vi "Process_LogEngine.vi"(8 "error in (no error)":errorcluster, 9 "start process sync notifier":refnum<notifier>, 11 "LogEngine":refnum<class "LogEngine.lvclass">) -> (0 "error out":errorcluster)   [LabVIEW 2022 SP3, in "LogEngine.lvclass"]
doc: "Developed by Kevin Thompson\nkevin@thompsonengineering.net\n\nCopyright 2018-2020\nThompson Engineering, LLC"
uses:
  LogEngine.lvclass
  LogEngine.lvclass/LogEngine.ctl
  Support/DataQueues/DataQueues.lvclass
  Support/DataQueues/DataTypes/Analog DataSet MultiRow & ChanNames--cluster.ctl
  Support/DataQueues/DataTypes/Analog DataSet MultiRow & ChanNames--QRef.ctl
  Data Types/DAQ Q & TaskName--cluster.ctl
  Support/DataQueues/DataTypes/DataQ SelectType--enum.ctl
  Data Types/TD Logger State--enum.ctl
  Data Types/AsyncCmd_LogEngine--enum.ctl
  Data Types/TD Logger State Data--cluster.ctl
  Ichor_Common/Lib/ErrorHandler/ErrorHandler.lvclass
  <vilib>/TELLC/SMQ/Add States to Queue using MultiLine String with vData.vi
  DAQ/DAQ.lvclass
  Sequencer/Sequencer.lvclass
  Data Types/TD LogEngine LocalSMData--cluster.ctl
  DataTypes/SessionSettings--cluster.ctl
  Data Types/LogHeaderData--cluster.ctl
  Application/Application.lvclass
  Sequencer/DataTypes/LoadSeqStatus--enum.ctl
  DAQ/DataTypes/AsyncMsg_DAQ--enum.ctl
  DAQ/DataTypes/TD AI InstSettings--cluster.ctl
  Data Types/TD LogEngine Settings--cluster.ctl
  Sequencer/DataTypes/LoadSeqStatus EvData--cluster.ctl
panel:
  in  "localData":cluster{"Msg":string, "vData":variant}
  in  "Stop Process":bool
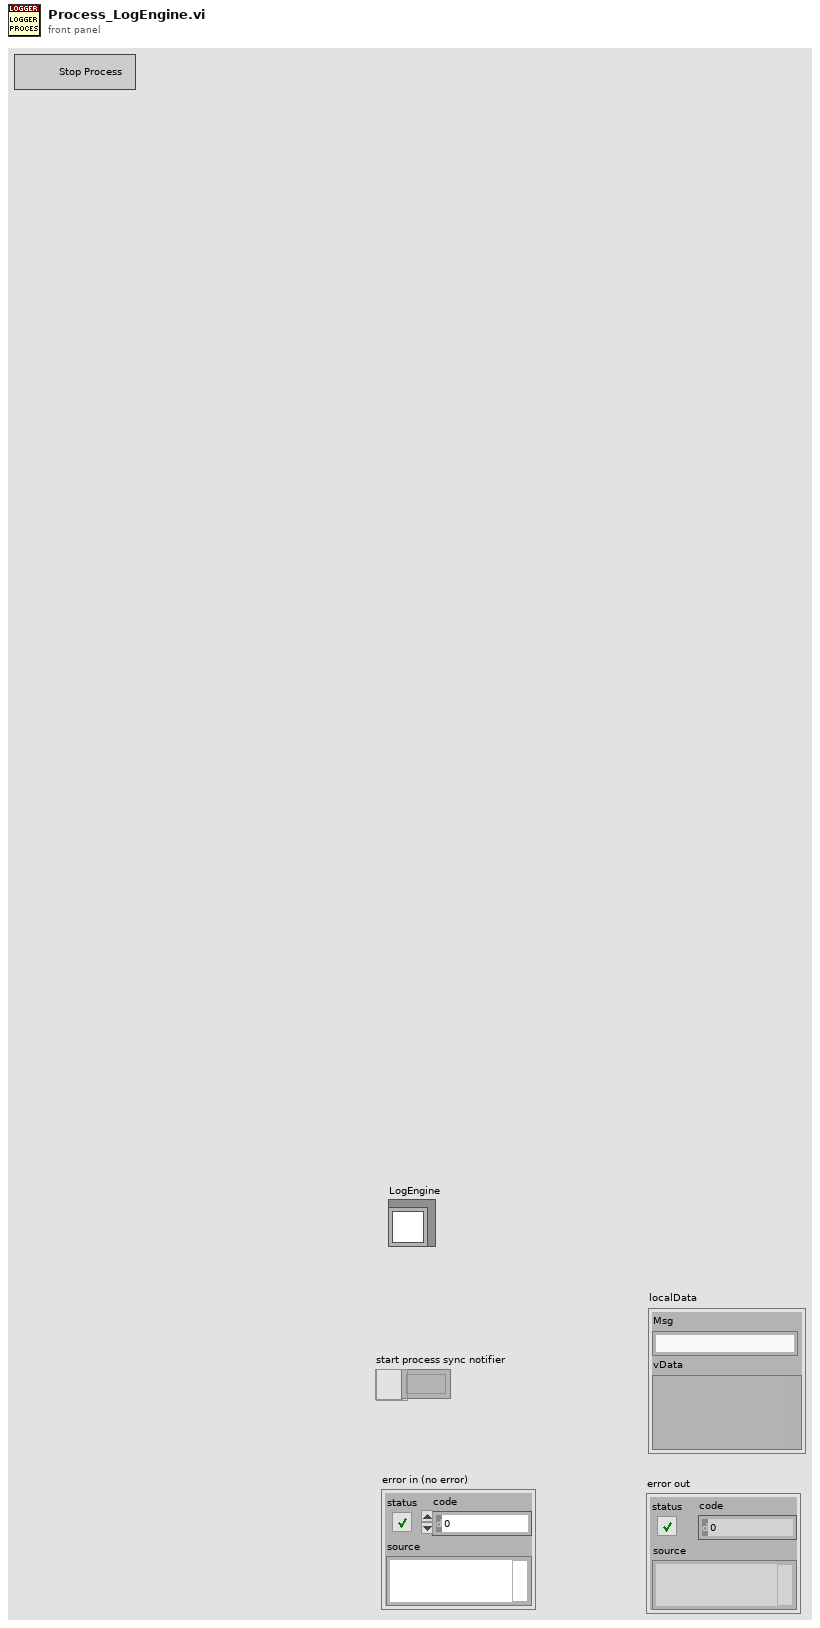
[diagram p1: front panel]
types:
  T1 = typedef "LogEngine.lvclass/TD LogEngine LocalSMData--cluster.ctl" = cluster{"Logging":bool, "tdms fileref":refnum<k34>, "Sequence File Path":string, "DAQ RawData Q []":T2[], "SMQ":refnum<queue>, "Core":cluster{"Current VI Ref":refnum<vi>, "process sync notifier":refnum<notifier>}, "quitting":bool, "Self Reference":refnum<class "LogEngine.lvclass">, "DAQ":refnum<class "DAQ.lvclass">, "TDMS file pathname":path, "Sequencer":refnum<class "Sequencer.lvclass">, "LogHeaderData":T4, "Application":refnum<class "Application.lvclass">, "dt(s)":dbl, "LogFile pathname":path, "LogEngine Settings":T6, "LogFile folder":path, "TDMS folder":path, "Logger State Data":T7, "TDMSLogging":bool, "HeaderStr Created?":bool, "TDMS SMQ":refnum<queue>, "StatusStr Ref":refnum<vi>, "Sampling dt(s)":dbl}
  T2 = typedef "LogEngine.lvclass/DAQ Q & TaskName--cluster.ctl" = cluster{"TaskName":string, "DAQ RawData Q":T3}
  T3 = typedef "DataQueues.lvclass/Analog DataSet MultiRow & ChanNames--QRef.ctl" = refnum<queue>
  T4 = typedef "LogEngine.lvclass/LogHeaderData--cluster.ctl" = cluster{"SessionSettings":T5, "SequenceFile":string, "Curr_WeldCount":i32, "AI TaskName":string, "SamplingRate":dbl, "SamplesPerAcq":i32}
  T5 = typedef "SessionSettings--cluster.ctl" = cluster{"Job_ID":string, "Operator_ID":string, "Station_ID":string, "Job_Description":string}
  T6 = typedef "LogEngine.lvclass/TD LogEngine Settings--cluster.ctl" = cluster{"placeholder":string, "LogWriteIntv (ms)":u32, "LogFile folder name":string, "TDMS folder name":string}
  T7 = typedef "LogEngine.lvclass/TD Logger State Data--cluster.ctl" = cluster{"Logger State":T8, "TDMS Logging State":T8, "LogFile path":path, "TDMS File path":path, "vData":variant}
  T8 = typedef "LogEngine.lvclass/TD Logger State--enum.ctl" = enum16{"Unknown", "Logging", "NotLogging", "Error"}
  T9 = typedef "DataQueues.lvclass/DataQ SelectType--enum.ctl" = enum16{"MainProcess", "LogEngine", "LocalDAQThread"}
  T10 = typedef "TD Pathnames--cluster.ctl" = cluster{"RunTimeSys?":bool, "AppFolder":path, "ExecutablePath":path, "ConfigFolder":path, "DataLogFolder":path, "SystemLogFolder":path, "SeqFolder":path, "MainStartupPathname":path, "MainUIPathname":path, "SystemEventsFile":path, "SeqEventsFile":path, "Config SettingsFile":path, "DAQ IOConfigFile":path, "SystemSimulation":bool}
  T11 = typedef "Sequencer.lvclass/LoadSeqStatus EvData--cluster.ctl" = cluster{"Time Stamp":timestamp, "OLD Status":T12, "NEW Status":T12}
  T12 = typedef "Sequencer.lvclass/LoadSeqStatus--enum.ctl" = enum16{"Unknown", "InProgress", "Loaded", "Failed"}
  T13 = typedef "DAQ.lvclass/AsyncMsg_DAQ--enum.ctl" = enum16{"DAQ.SendAI_InstSettings"}
  T14 = typedef "LogEngine.lvclass/AsyncCmd_LogEngine--enum.ctl" = enum16{"LE.CreateLogFile", "LE.EnableLogging", "LE.OpenTDMS", "LE.CloseTDMS", "LE.StartTDMSLogging", "LE.StopTDMSLogging", "LE.AppendStrToLog", "LE.ClearLogFilePathname"}
  T15 = typedef "Application.lvclass/AsynMsg_Application--enum.ctl" = enum16{"Application.AppClassReference", "Application.RefreshSettings", "Application.SendSessionSettings"}
  T16 = typedef "LogEngine.lvclass/TD Obj Data_LogEngine.ctl" = cluster{"LogEngine Settings":T6, "Logger State Data":T7, "tdms fileref":refnum<k34>, "LogHeaderData":T4, "LogHeaderString":string}
  T17 = typedef "Sequencer.lvclass/AsynMsg_Sequencer--enum.ctl" = enum16{"Sequencer.LoadSeqStatusChg", "Sequencer.SeqExecStatusChg", "Sequencer.SeqStepChg"}
  T18 = typedef "DAQ.lvclass/TD AI InstSettings--cluster.ctl" = cluster{"DaqRate":dbl, "NumSamples":i32}
  T19 = cluster{"AI InstSettings":T18, "AI TaskName":string}
  T20 = cluster{"dup Directory Path":path, "dup Directory Path":path}
  T21 = typedef "DAQ.lvclass/TD AI Instrument Settings--cluster.ctl" = cluster{"Disable":bool, "AI TaskName":string, "AI InstSettings":T18, "SimAI Ranges":T22}
  T22 = typedef "DAQ.lvclass/TD SimAI Ranges--cluster.ctl" = cluster{"lo":dbl, "hi":dbl}
  T23 = typedef "LogEngine.lvclass/TD LogEngine PublicEvents--cluster.ctl" = cluster{"stop process":refnum<user-event>, "LogEngine.AsyncCmd Event":refnum<user-event>, "LogEngine.AsyncMsg Event":refnum<user-event>, "Logger StateChanged Event":refnum<user-event>}
  T24 = typedef "Application.lvclass/Public Events--cluster.ctl" = cluster{"Application.AsyncCmd Event":refnum<user-event>, "Application.AsyncMsg Event":refnum<user-event>, "stop process":refnum<user-event>, "Application.ControlStateChg Event":refnum<user-event>, "Application.RadialGraph Event":refnum<user-event>}
  T25 = typedef "Sequencer.lvclass/Public Events--cluster.ctl" = cluster{"Sequencer.AsyncCmd Event":refnum<user-event>, "Sequencer.AsyncMsg Event":refnum<user-event>, "stop process":refnum<user-event>}
  T26 = typedef "DAQ.lvclass/TD PublicEvents--cluster.ctl" = cluster{"DaqOutputCmd Ev":refnum<user-event>, "stop process":refnum<user-event>, "DAQ.AsyncCmd Event":refnum<user-event>, "DAQStateChanged Event":refnum<user-event>, "DAQ.AsyncMsg Event":refnum<user-event>}
  T27 = cluster{bool, "Logger State Data":T7, "LogFile pathname":path}
  T28 = enum16{"open", "open or create", "create or replace", "create", "open (read-only)"}
  T29 = cluster{bool, "Logger State Data":T7, "TDMS file pathname":path}
  T30 = cluster{string, cluster{bool, "Logger State Data":T7, "TDMS file pathname":path}}
  T31 = cluster{string, cluster{bool, "Logger State Data":T7, path}}
  T32 = cluster{"Actuator ID":string[], "Cap":dbl[], "DF":dbl[], "Parameter":string[], "Parameter label":string, "Notes":string}
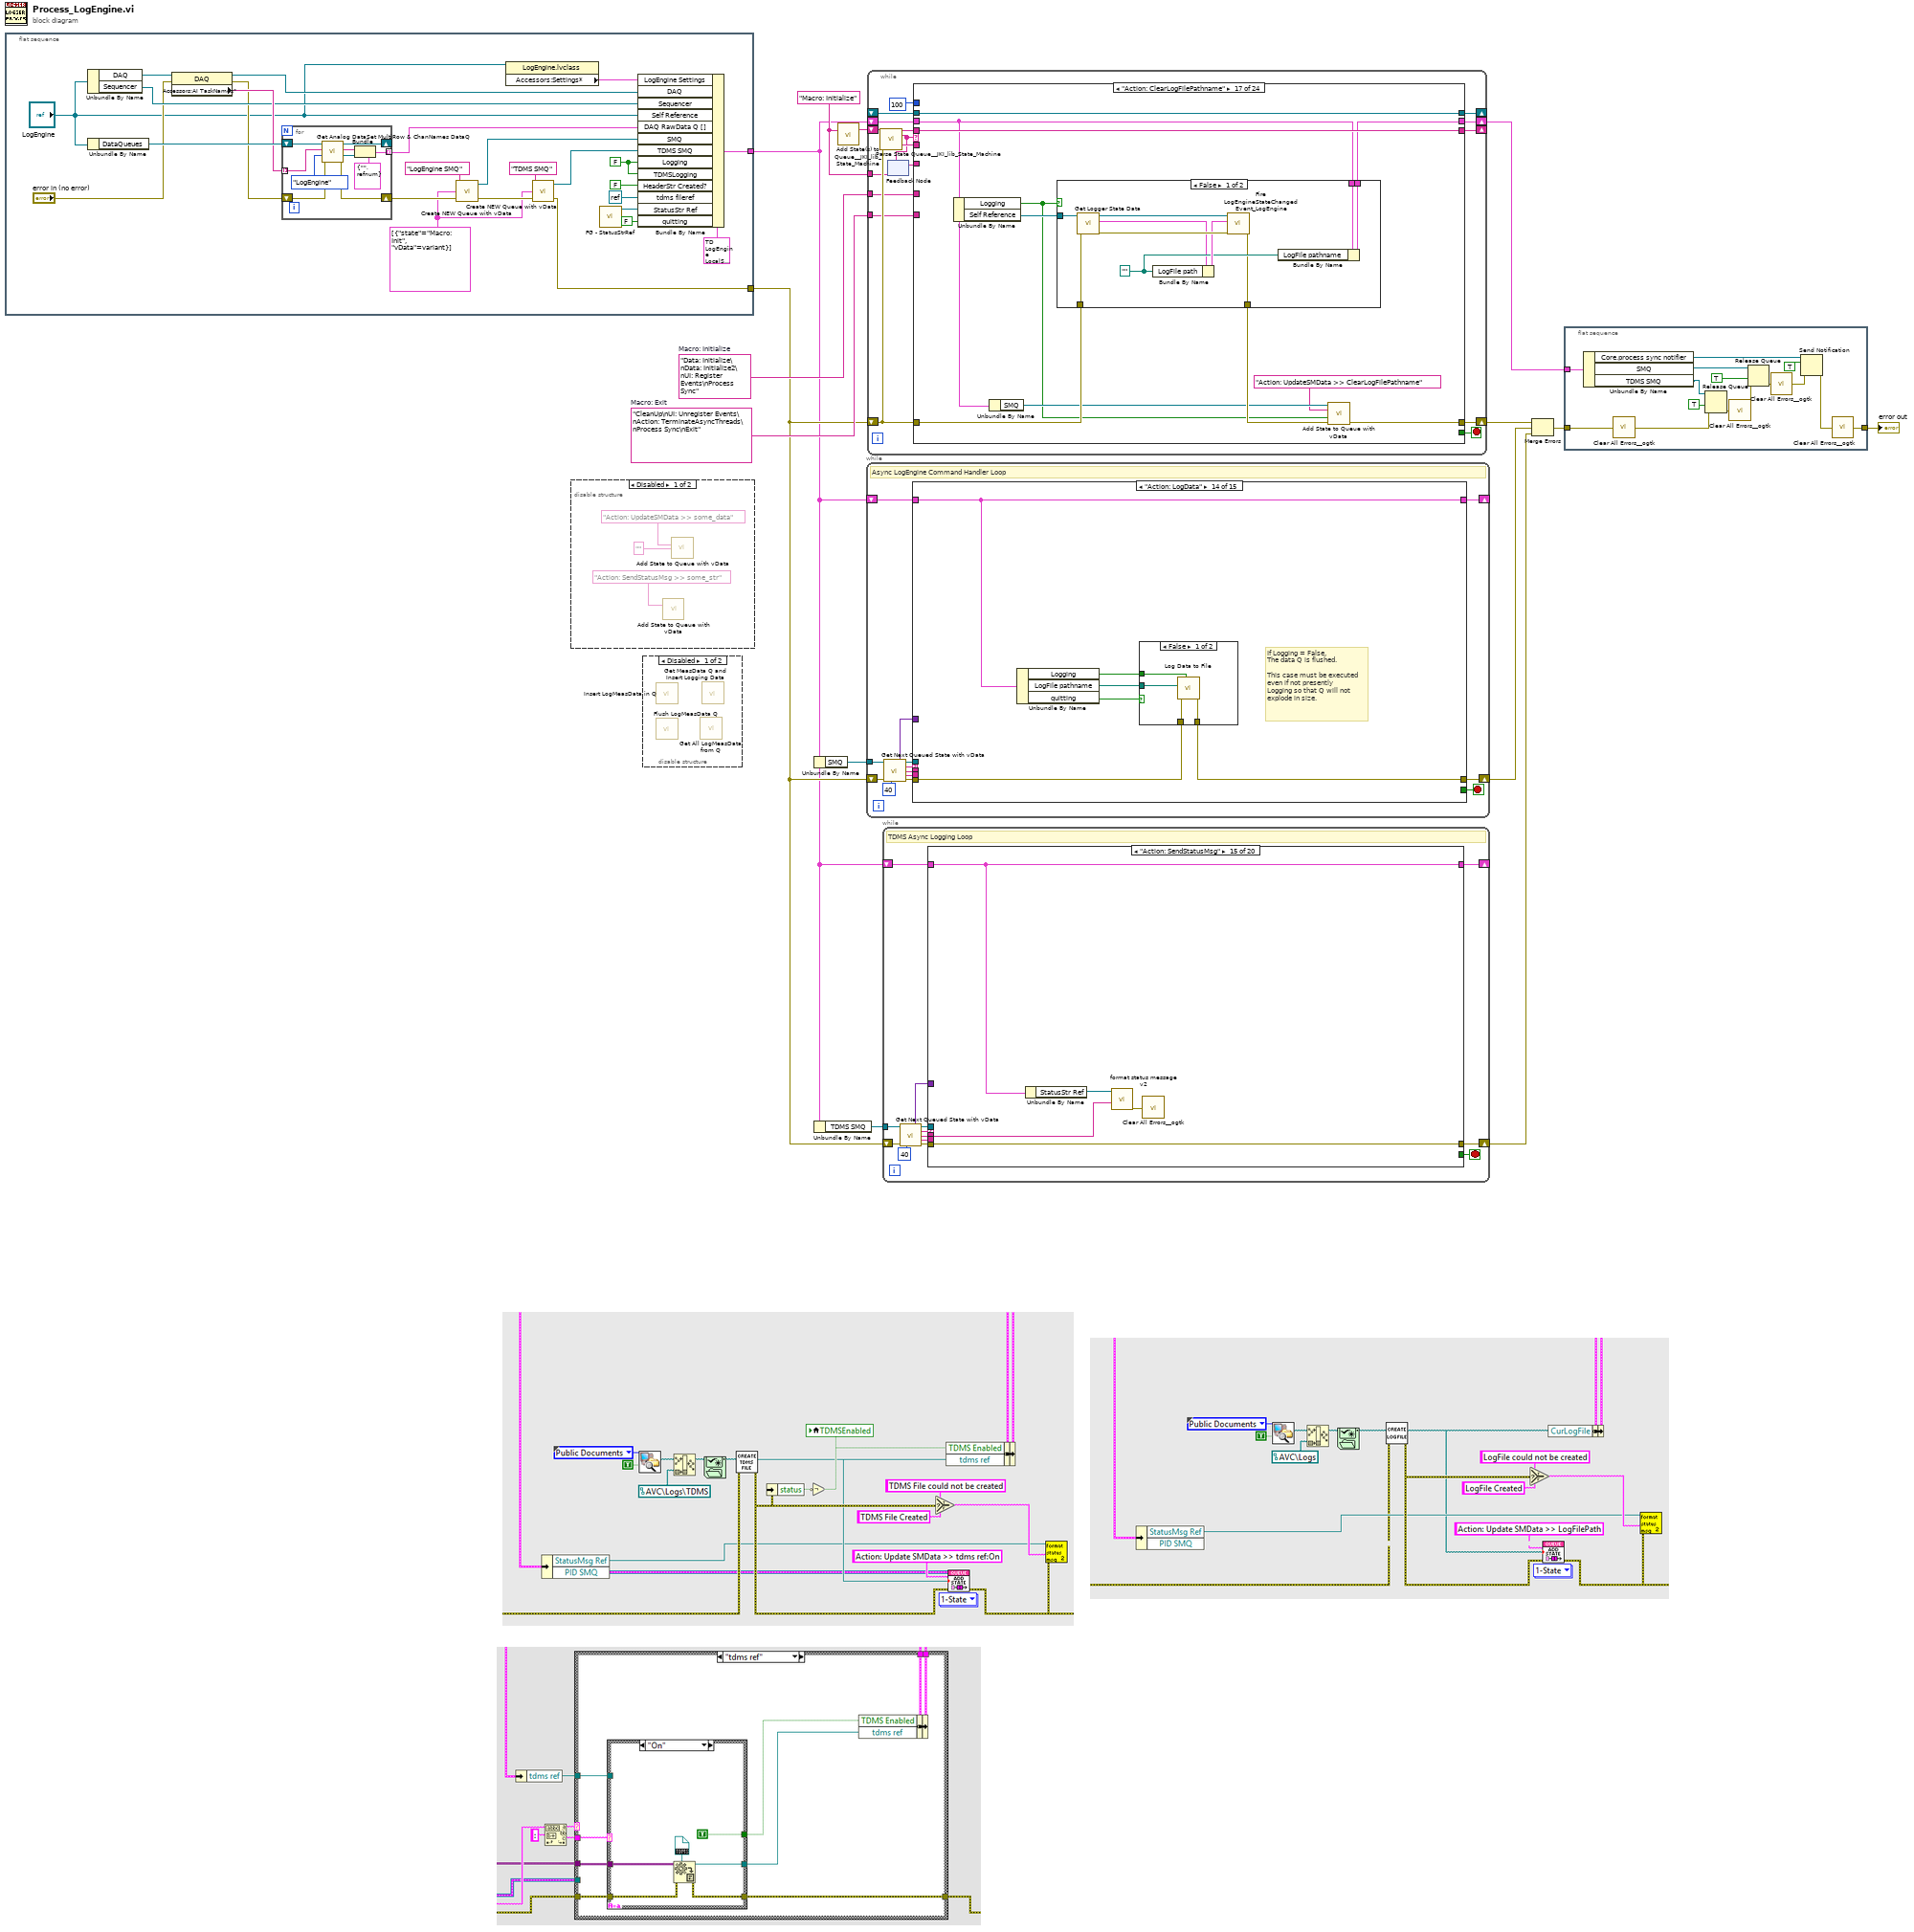
[diagram p0: block diagram]
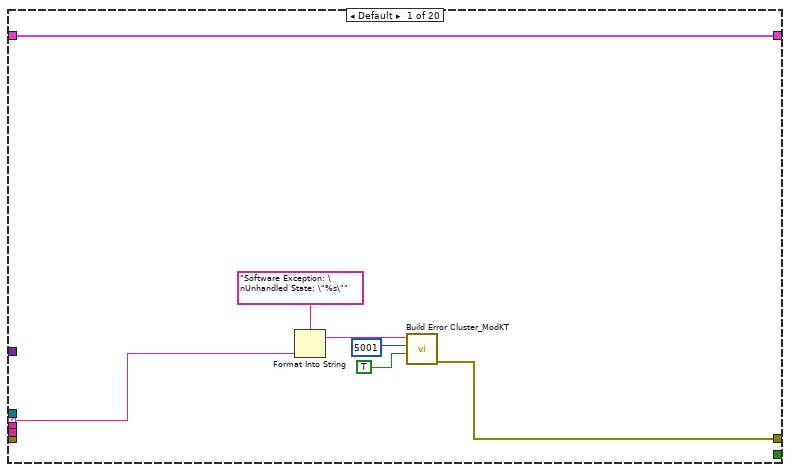
[diagram p2: hidden frame]
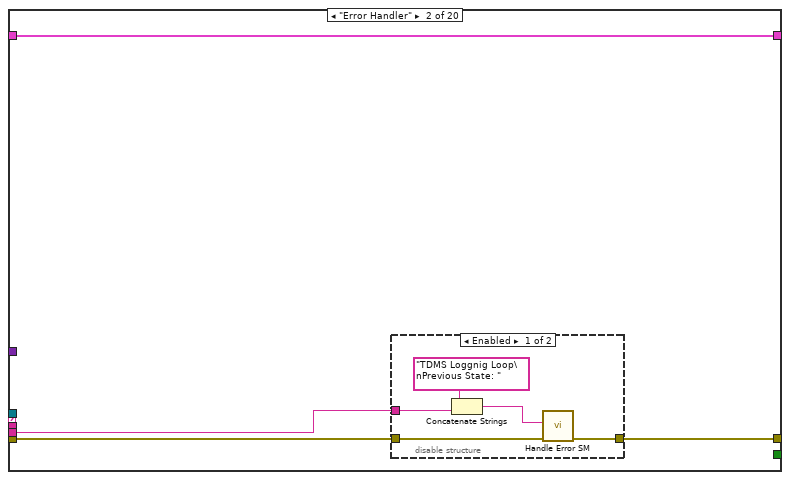
[diagram p3: hidden frame]
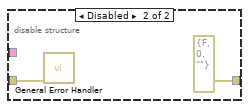
[diagram p4: hidden frame]
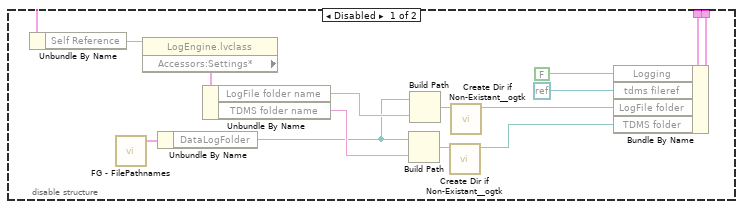
[diagram p6: hidden frame]
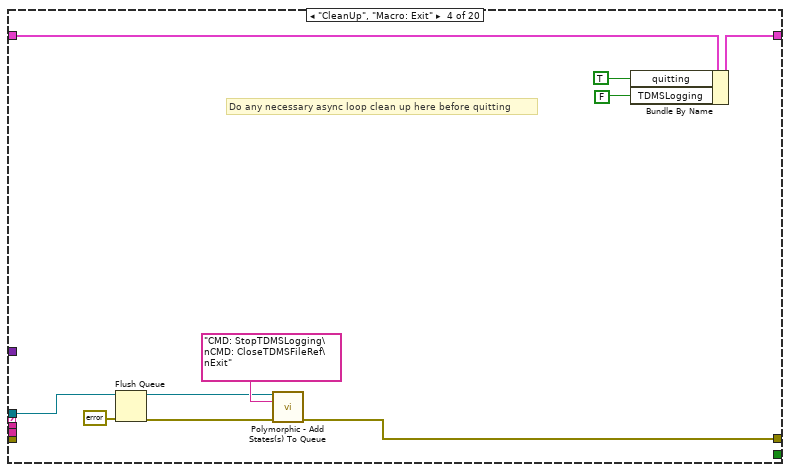
[diagram p7: hidden frame]
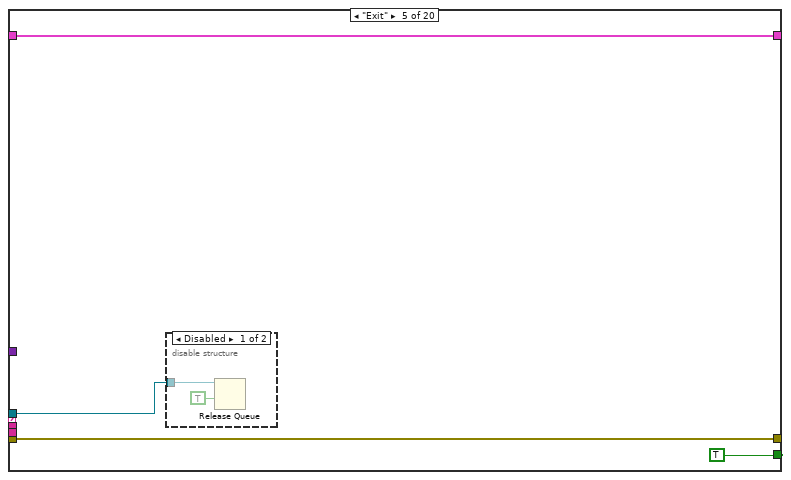
[diagram p8: hidden frame]
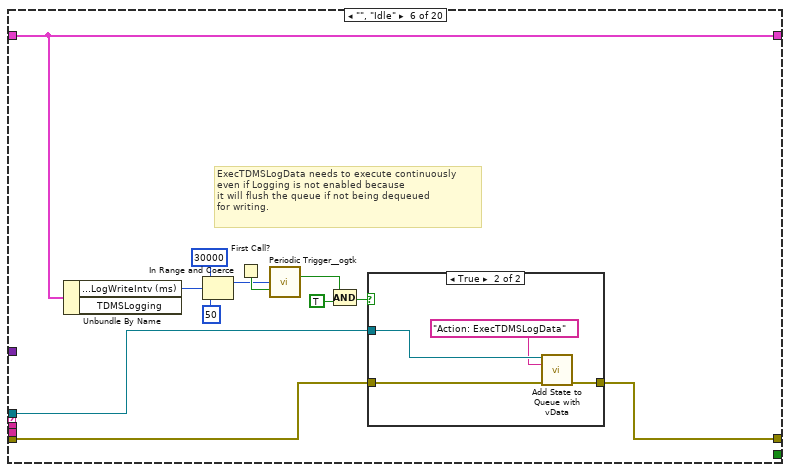
[diagram p10: hidden frame]
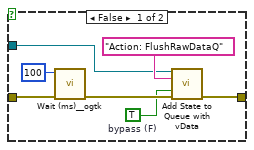
[diagram p11: hidden frame]
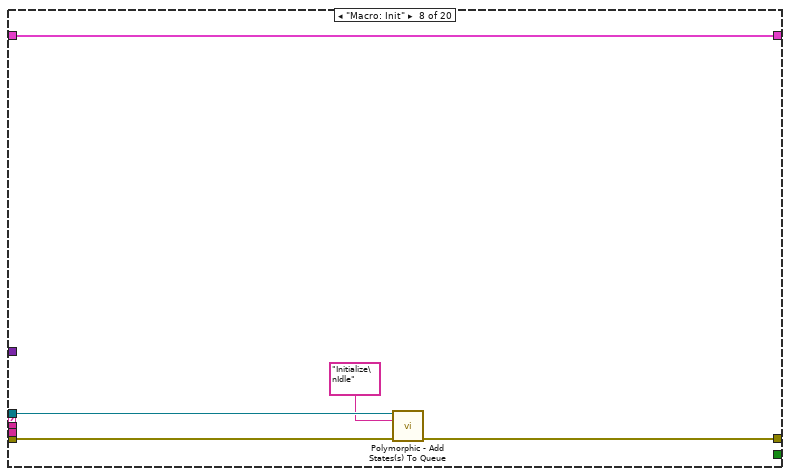
[diagram p13: hidden frame]
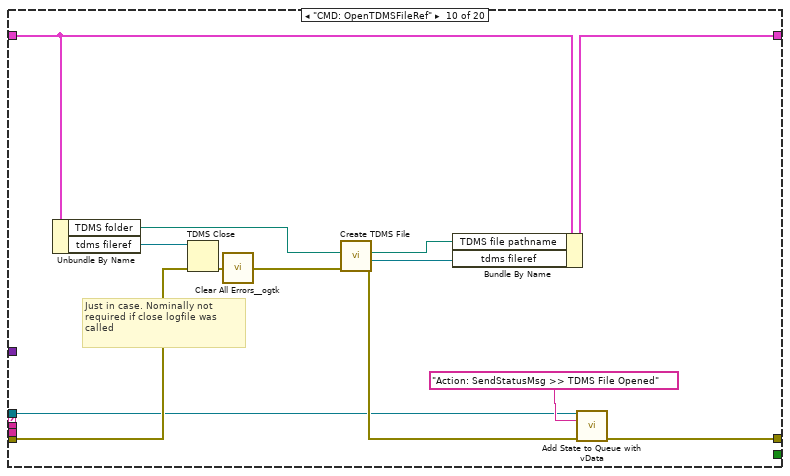
[diagram p15: hidden frame]
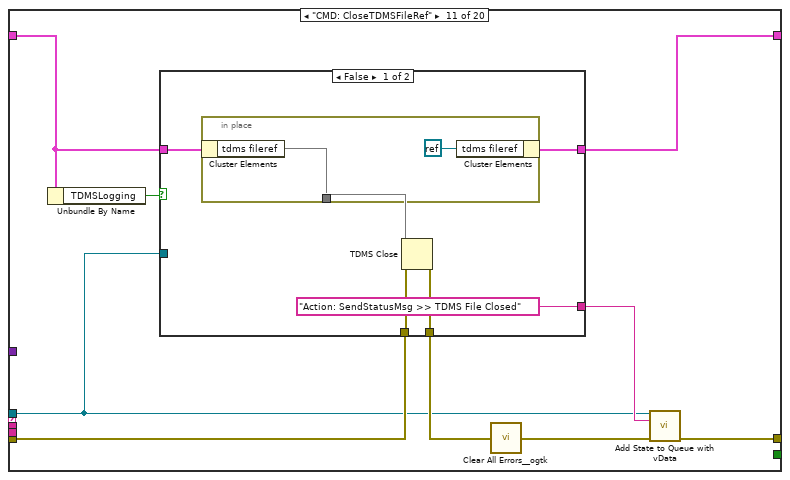
[diagram p16: hidden frame]
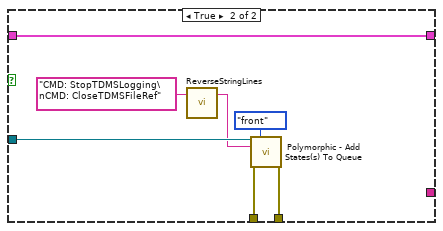
[diagram p17: hidden frame]
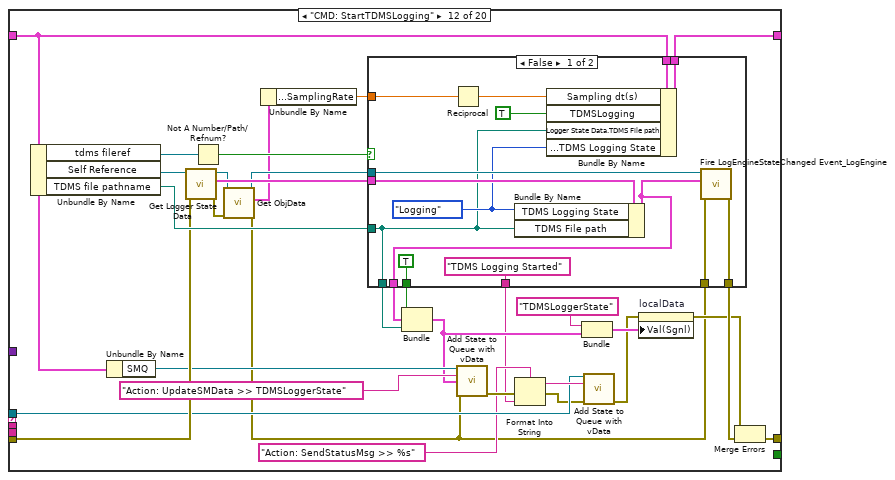
[diagram p18: hidden frame]
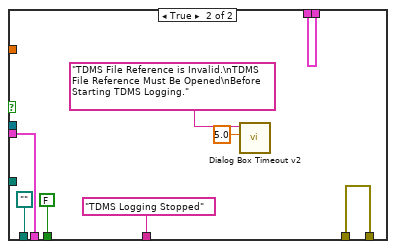
[diagram p19: hidden frame]
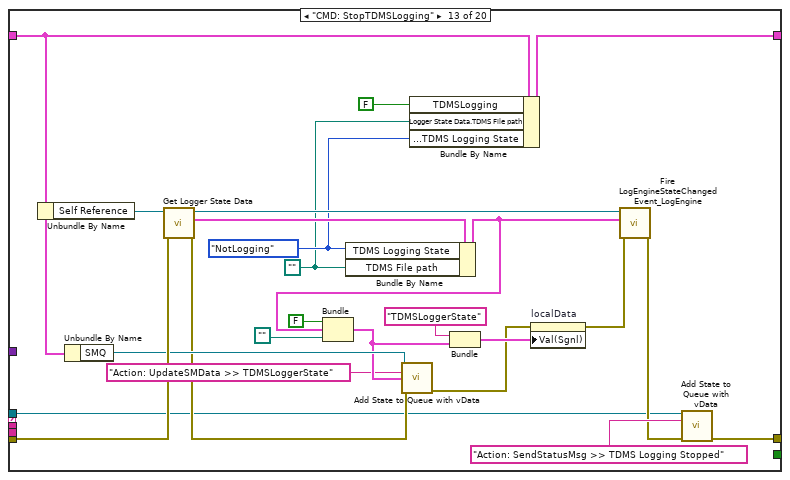
[diagram p20: hidden frame]
diagram:
  w13 = "Data: Initialize\nData: Initialize2\nUI: Register Events\nProcess Sync"  # Macro: Initialize
  w12 = "CleanUp\nUI: Unregister Events\nAction: TerminateAsyncThreads\nProcess Sync\nExit"  # Macro: Exit
  w8 = "Macro: Initialize"
  n1 = flat-sequence {
    tunnel: [w19] -> w7
    tunnel: [w33] -> w6
    frame #0 {
      w24 = FALSE
      w18 = cluster{"state":string, "vData":variant}[] [{"state"="Macro: Init", "vData"=variant}] ("Initial States")
      n2 = Unbundle By Name("LogEngine") -> ("DAQ"=w32:refnum<class "DAQ.lvclass">, "Sequencer"=w31:refnum<class "Sequencer.lvclass">)
      n3 = Unbundle By Name("LogEngine") -> ("DataQueues"=w37:refnum<class "DataQueues.lvclass">)
      n4 = property class="DAQ"(reference=w32, error in="error in (no error)") -> (reference out=w34:refnum<class "DAQ.lvclass">, error out=w28:errorcluster, "Accessors:AI TaskNames*"=w36:string[])
      n5 = for {
        shift-right: [w48] -> _
        shift-left: w37 -> [w49]
        tunnel: w36 -> [w47] mode=indexing
        tunnel: [w42] -> w35 mode=indexing
        shift-right: [w40] -> w30
        shift-left: w28 -> [w46]
        n6 = call "Get Analog DataSet MultiRow & ChanNames DataQ.vi"("error in (no error)"=w46, "Select"=DataQ_SelectType--enum."LogEngine", "TaskName"=w47, "DataQueues in"=w49) -> ("error out"=w40:errorcluster, "Analog DataSet MultiRow & ChanNames QRef"=w43:T3, "TaskName out"=w44:string, "DataQueues out"=w48:refnum<class "DataQueues.lvclass">)  [unwired: 3 in, 1 out]
        n7 = Bundle(cluster=T2 {"TaskName"="", "DAQ RawData Q"=refnum} ("Data Q & TaskName"), "TaskName"=w44, "DAQ RawData Q"=w43) -> (w42:T2)
      }
      n8 = call <vilib>:"Create NEW Queue with vData.vi"("error in (no error)"=w30, "Initial States"=w18, "Name (SMQ)"="LogEngine SMQ") -> ("error out"=w20:errorcluster, "queue out"=w38:refnum<queue>)  [unwired: 1 in]
      n9 = property class="LogEngine.lvclass"(reference="LogEngine") -> ("Accessors:Settings*"=w25:T6)  [unwired: 1 in, 2 out]
      n10 = call <vilib>:"Create NEW Queue with vData.vi"("error in (no error)"=w20, "Initial States"=w18, "Name (SMQ)"="TDMS SMQ") -> ("error out"=w19:errorcluster, "queue out"=w17:refnum<queue>)  [unwired: 1 in]
      n11 = call "FG - StatusStrRef.vi"() -> ("StatusStr Ref out"=w16:refnum<vi>)  [unwired: 9 in, 1 out]
      n12 = Bundle By Name(cluster=T1 {"Logging"=FALSE, "tdms fileref"=refnum, "Sequence File Path"="", "DAQ RawData Q []"=[], "SMQ"=refnum, "Core"={"Current VI Ref"=refnum, "process sync notifier"=refnum}, "quitting"=FALSE, "Self Reference"=refnum, "DAQ"=refnum, "TDMS file pathname"=path "", "Sequencer"=refnum, "LogHeaderData"={"SessionSettings"={"Job_ID"="", "Operator_ID"="", "Station_ID"="", "Job_Description"=""}, "SequenceFile"="", "Curr_WeldCount"=0, "AI TaskName"="", "SamplingRate"=0.0, "SamplesPerAcq"=0}, "Application"=refnum, "dt(s)"=0.0, "LogFile pathname"=path "", "LogEngine Settings"={"placeholder"="", "LogWriteIntv (ms)"=0, "LogFile folder name"="", "TDMS folder name"=""}, "LogFile folder"=path "", "TDMS folder"=path "", "Logger State Data"={"Logger State"=enum."Unknown", "TDMS Logging State"=enum."Unknown", "LogFile path"=path "", "TDMS File path"=path "", "vData"=variant}, "TDMSLogging"=FALSE, "HeaderStr Created?"=FALSE, "TDMS SMQ"=refnum, "StatusStr Ref"=refnum, "Sampling dt(s)"=0.0} ("TDMS LocalSMData"), "LogEngine Settings"=w25, "DAQ"=w34, "Sequencer"=w31, "Self Reference"="LogEngine", "DAQ RawData Q []"=w35, "SMQ"=w38, "TDMS SMQ"=w17, "Logging"=w24, "TDMSLogging"=w24, "HeaderStr Created?"=FALSE, "tdms fileref"=refnum<k0> refnum, "StatusStr Ref"=w16, "quitting"=FALSE) -> (w33:T1)
    }
  }
  n13 = disable-structure shown="Disabled" {
    frame Disabled {
      n14 = call <vilib>:"Add State to Queue with vData.vi"("state in"="Action: SendStatusMsg >> some_str") -> ()  [unwired: 11 in, 4 out]
      n15 = call <vilib>:"Add State to Queue with vData.vi"("state in"="Action: UpdateSMData >> some_data", "vData (\"\")"="") -> ()  [unwired: 10 in, 4 out]
    }
    frame Enabled {
    }
  }
  n16 = disable-structure shown="Disabled" {
    frame Disabled {
      n17 = call "Insert LogMeasData in Q.vi"() -> ()  [unwired: 9 in, 3 out]
      n18 = call "Flush LogMeasData Q.vi"() -> ()  [unwired: 9 in, 3 out]
      n19 = call "Get All LogMeasData from Q.vi"() -> ()  [unwired: 8 in, 4 out]
      n20 = call "Get MeasData Q and Insert Logging Data.vi"() -> ()  [unwired: 9 in, 3 out]
    }
    frame Enabled {
    }
  }
  n21 = Unbundle By Name(w6) -> ("SMQ"=w9:refnum<queue>)
  n22 = Unbundle By Name(w6) -> ("TDMS SMQ"=w5:refnum<queue>)
  n23 = call <vilib>:"Add State(s) to Queue__JKI_lib_State_Machine.vi"("State(s) in (\"\")"=w8) -> ("States Out"=w14:string)  [unwired: 14 in]
  n24 = while {
    shift-right: [w54] -> _
    shift-left: w6 -> [w55]
    tunnel: w9 -> [w65]
    shift-right: [w57] -> w10
    shift-left: w7 -> [w59]
    stop <- w56 stop-if-true
    # "Async LogEngine Command Handler Loop"
    n25 = call <vilib>:"Get Next Queued State with vData.vi"("queue in"=w65, "error in (no error)"=w59, "timeout (100)"=40) -> ("vData out"=w60:variant, "queue out"=w63:refnum<queue>, "Next State"=w64:string, "queued msg"=w62:string, "Prev State"=w61:string, "error out"=w58:errorcluster)  [unwired: 6 in, 1 out]
    n26 = case shown="\"Action: LogData\"" w64 {
      tunnel: w58 -> [_ w74 w85 _ w112 w127 w146 w151 w153 w155 w164 w171 w173 w229 w239]
      tunnel: w63 -> [_ _ _ w111 w113 w128 _ w148 _ _ _ _ _ _ _]
      tunnel: w62 -> [_ _ _ _ _ _ _ _ _ _ _ w167 w176 _ _]
      selector: w64 -> [w66 _ _ _ _ _ _ _ _ _ _ _ _ _ _]
      tunnel: w61 -> [_ w73 _ _ _ _ _ _ _ _ _ _ _ _ _]
      tunnel: w60 -> [_ _ _ _ _ _ _ _ _ _ w165 _ w177 _ _]
      tunnel: [w67 w75 w85 w106 w112 w126 w146 w149 w153 w155 w157 w171 w172 w228 w239] -> w57
      tunnel: [_ _ _ _ TRUE _ _ _ _ _ _ _ _ _ _] -> w56
      tunnel: w55 -> [w72 w76 w84 w105 w114 w129 w145 w150 w152 w154 w166 w168 w175 w232 w238]
      tunnel: [w72 w76 w86 w104 w114 w129 w145 w150 w152 w154 w166 w168 w174 w232 w238] -> w54
      frame Default {
        n27 = Format Into String(format string="Software Exception: \nUnhandled State: \"%s\"", w66) -> (resulting string=w69:string)  [unwired: 2 in, 1 out]
        n28 = call <vilib>:"Build Error Cluster_ModKT .vi"("Prepend String (\"\")"=w69, "code"=5001, "error? (F)"=TRUE ("error?")) -> ("error out"=w67:errorcluster)  [unwired: 4 in, 1 out]
      }
      frame "Error Handler" {
        n29 = disable-structure shown="Enabled" {
          disable-tunnel: [w79 errorcluster {"status"=FALSE, "code"=0, "source"=""} ("error constant")] -> w75
          disable-tunnel: w74 -> [w78 w82]
          disable-tunnel: w73 -> [w77 _]
          frame Enabled {
            n30 = Concatenate Strings("LogEngine Logging Loop\nPrevious State: ", w77) -> (w80:string)
            n31 = call "Handle Error SM.vi"("error in (no error)"=w78, "CustomMessage"=w80) -> ("error out"=w79:errorcluster)  [unwired: 7 in, 2 out]
          }
          frame Disabled {
            n32 = call <vilib>:"General Error Handler.vi"("error in (no error)"=w82) -> ()  [unwired: 10 in, 5 out]
          }
        }
      }
      frame "Initialize" {
        n33 = disable-structure shown="Enabled" {
          disable-tunnel: [w100 w101] -> w86
          disable-tunnel: w84 -> [w96 w101]
          frame Disabled {
            n34 = Unbundle By Name(w96) -> ("Self Reference"=w95:refnum<class "LogEngine.lvclass">)
            n35 = call "FG - FilePathnames.vi"() -> ("FilePaths out"=w97:T10)  [unwired: 4 in, 1 out]
            n36 = property class="LogEngine.lvclass"(reference=w95) -> ("Accessors:Settings*"=w94:T6)  [unwired: 1 in, 2 out]
            n37 = Unbundle By Name(w97) -> ("DataLogFolder"=w89:path)
            n38 = Unbundle By Name(w94) -> ("LogFile folder name"=w92:string, "TDMS folder name"=w90:string)
            n39 = Build Path(base path=w89, name or relative path=w90) -> (appended path=w91:path)
            n40 = Build Path(base path=w89, name or relative path=w92) -> (appended path=w93:path)
            n41 = call <userlib>:"Create Dir if Non-Existant__ogtk.vi"("Directory Path"=w91) -> ("dup Directory Path"=w87:path)  [unwired: 8 in, 2 out]
            n42 = call <userlib>:"Create Dir if Non-Existant__ogtk.vi"("Directory Path"=w93) -> ("dup Directory Path"=w88:path)  [unwired: 8 in, 2 out]
            n43 = Bundle By Name(cluster=w96, "Logging"=FALSE, "tdms fileref"=refnum<k0> refnum, "LogFile folder"=w88, "TDMS folder"=w87) -> (w100:T1)
          }
          frame Enabled {
          }
        }
      }
      frame "CleanUp", "Macro: Exit" {
        # "Do any necessary async loop clean up here before quitting"
        n44 = Flush Queue(queue=w111, error in (no error)=errorcluster {"status"=FALSE, "code"=0, "source"=""}) -> (queue out=w107:refnum<queue>, error out=w109:errorcluster)  [unwired: 1 out]
        n45 = call-poly <vilib>:"Polymorphic - Add States(s) To Queue.vi"("queue in"=w107, "states in"="Exit", "error in"=w109) -> ("error out"=w106:errorcluster)  [unwired: 10 in, 2 out]
        n46 = Bundle By Name(cluster=w105, "Logging"=FALSE, "quitting"=TRUE) -> (w104:T1)
      }
      frame "Exit" {
        n47 = disable-structure shown="Disabled" {
          disable-tunnel: w113 -> [w116 _]
          frame Disabled {
            n48 = Release Queue(queue=w116, force destroy? (F)=TRUE) -> ()  [unwired: 1 in, 3 out]
          }
          frame Enabled {
          }
        }
      }
      frame "", "Idle" {
        # "LogData needs to execute continuously\neven if Logging is not enabled because\nit will flush the queue if not being dequeued\nfor writing."
        n49 = Unbundle By Name(w129) -> ("LogEngine Settings.LogWriteIntv (ms)"=w120:u32)  [unwired: 1 out]
        n50 = In Range and Coerce(upper limit=u32 30000, x=w120, lower limit=u32 50) -> (coerced(x)=w121:u32)  [unwired: 1 out]
        n51 = First Call?() -> (First Call?: T/F=w125:bool)
        n52 = call <userlib>:"Periodic Trigger__ogtk.vi"("time (ms)"=w121, "reset"=w125) -> ("Triggered"=w124:bool)  [unwired: 11 in, 2 out]
        n53 = Compound Arithmetic op=AND(w124, TRUE ("value")) -> (w123:bool)
        n54 = case shown="True" w123 {
          tunnel: w128 -> [w130 w144]
          tunnel: w127 -> [w133 w142]
          tunnel: [w131 w141] -> w126
          frame False {
            n55 = call <userlib>:"Wait (ms)__ogtk.vi"("error in (no error)"=w133, "milliseconds to wait"=u32 100) -> ("error out"=w132:errorcluster)  [unwired: 8 in, 1 out]
            n56 = disable-structure shown="Enabled" {
              disable-tunnel: w132 -> [w138 w140]
              disable-tunnel: [w137 w140] -> w131
              disable-tunnel: w130 -> [w136 _]
              frame Disabled {
                n57 = call <vilib>:"Add State to Queue with vData.vi"("queue in"=w136, "state in"="Action: FlushRawDataQ", "bypass (F)"=TRUE, "error in"=w138) -> ("error out"=w137:errorcluster)  [unwired: 8 in, 3 out]
              }
              frame Enabled {
              }
            }
          }
          frame True {
            n58 = call <vilib>:"Add State to Queue with vData.vi"("queue in"=w144, "state in"="Action: LogData", "error in"=w142) -> ("error out"=w141:errorcluster)  [unwired: 9 in, 3 out]
          }
        }
      }
      frame "------ Macro ------" {
      }
      frame "Macro: Init" {
        n59 = call-poly <vilib>:"Polymorphic - Add States(s) To Queue.vi"("queue in"=w148, "states in"="Initialize\nIdle", "error in"=w151) -> ("error out"=w149:errorcluster)  [unwired: 10 in, 2 out]
      }
      frame "------ Cmd ------" {
      }
      frame "------ Action ------" {
      }
      frame "Action: AppendStringToLog" {
        n60 = Variant To Data(error in=w164, type="", Variant=w165) -> (data=w158:string, error out=w163:errorcluster)
        n61 = Unbundle By Name(w166) -> ("LogFile pathname"=w159:path)  [unwired: 1 out]
        n62 = call <vilib>:"Write Characters To File mod2KT.vi"("append to file? (new file:F)"=TRUE, "advisory dialog? (display:T)"=FALSE, "character string"=w158, "file path (dialog if empty)"=w159) -> ("error out"=w156:errorcluster)  [unwired: 2 in, 1 out]
        n63 = Merge Errors(w156, w163) -> (w157:errorcluster)
      }
      frame "Action: SendStatusMsg" {
        n64 = Unbundle By Name(w168) -> ("StatusStr Ref"=w169:refnum<vi>)
        n65 = call <vilib>:"format status message v2.vi"("status msg"=w167, "Str Refnum"=w169) -> ("error out"=w170:errorcluster)  [unwired: 5 in, 4 out]
        n66 = call <userlib>:"Clear All Errors__ogtk.vi"("Error In"=w170) -> ()  [unwired: 3 in, 1 out]
      }
      frame "Action: UpdateSMData" {
        n67 = case shown="\"ClearLogFilePathname\"" w176 {
          tunnel: w177 -> [_ w192 _ w206 w219 w226]
          tunnel: w173 -> [w178 w191 w194 w205 w218 w225]
          tunnel: w175 -> [w179 w190 w196 w204 w217 w224]
          tunnel: [w179 w189 w195 w203 w216 w223] -> w174
          tunnel: [w178 w188 w194 w202 w215 w221] -> w172
          frame Default {
          }
          frame "LoggerState" {
            n68 = Bundle(FALSE, "Logger State Data"=T7 {"Logger State"=enum."Unknown", "TDMS Logging State"=enum."Unknown", "LogFile path"=path "", "TDMS File path"=path "", "vData"=variant}, path "") -> (w185:cluster{bool, "Logger State Data":T7, path})  [unwired: 1 in]
            n69 = Variant To Data(error in=w191, type=w185, Variant=w192) -> (data=w184:cluster{bool, "Logger State Data":T7, path}, error out=w188:errorcluster)
            n70 = Unbundle(w184) -> (w183:bool, "Logger State Data"=w182:T7, w180:path)
            n71 = Bundle By Name(cluster=w190, "Logging"=w183, "Logger State Data"=w182, "LogFile pathname"=w180) -> (w189:T1)
          }
          frame "ClearLogFilePathname" {
            n72 = Bundle By Name(cluster=w196, "LogFile pathname"=path "") -> (w195:T1)
          }
          frame "Log&TDMS_Folders" {
            w197 = path ""
            n73 = Bundle(w197, w197) -> (w201:cluster{path, path})  [unwired: 1 in]
            n74 = Variant To Data(error in=w205, type=w201, Variant=w206) -> (data=w200:cluster{path, path}, error out=w202:errorcluster)
            n75 = Unbundle(w200) -> (w199:path, w198:path)
            n76 = Bundle By Name(cluster=w204, "LogFile folder"=w199, "TDMS folder"=w198) -> (w203:T1)
          }
          frame "TDMSLoggerState" {
            n77 = Bundle(FALSE, "Logger State Data"=T7 {"Logger State"=enum."Unknown", "TDMS Logging State"=enum."Unknown", "LogFile path"=path "", "TDMS File path"=path "", "vData"=variant}, path "") -> (w212:cluster{bool, "Logger State Data":T7, path})  [unwired: 1 in]
            n78 = Variant To Data(error in=w218, type=w212, Variant=w219) -> (data=w211:cluster{bool, "Logger State Data":T7, path}, error out=w215:errorcluster)
            n79 = Unbundle(w211) -> (w210:bool, "Logger State Data"=w209:T7, w207:path)
            n80 = Bundle By Name(cluster=w217, "TDMSLogging"=w210, "Logger State Data"=w209, "TDMS file pathname"=w207) -> (w216:T1)
          }
          frame "SessionSettings" {
            n81 = Variant To Data(error in=w225, type=T5 {"Job_ID"="", "Operator_ID"="", "Station_ID"="", "Job_Description"=""} ("Session Settings"), Variant=w226) -> (data=w222:T5, error out=w221:errorcluster)
            n82 = Bundle By Name(cluster=w224, "LogHeaderData.SessionSettings"=w222) -> (w223:T1)
          }
        }
      }
      frame "Action: LogData" {
        # "If Logging = False,\nThe data Q is flushed.\n\nThis case must be executed\neven if not presently\nLogging so that Q will not\nexplode in size."
        n83 = Unbundle By Name(w232) -> ("Logging"=w231:bool, "LogFile pathname"=w230:path, "quitting"=w227:bool)
        n84 = case shown="False" w227 {
          tunnel: w231 -> [w236 _]
          tunnel: w230 -> [w235 _]
          tunnel: w229 -> [w234 w237]
          tunnel: [w233 w237] -> w228
          frame False {
            n85 = call "Log Data to File.vi"("WriteLogFile (T)"=w236, "error in (no error)"=w234, "Path"=w235) -> ("error out"=w233:errorcluster)  [unwired: 7 in, 1 out]
          }
          frame True {
          }
        }
      }
      frame "----------- HOLD --------------" {
      }
    }
  }
  n86 = while {
    shift-right: [w250] -> w1
    shift-left: w6 -> [w249]
    shift-right: [w253] -> w11
    shift-left: w7 -> [w248]
    shift-right: [w252] -> _
    shift-left: w14 -> [w254]
    shift-right: [w246] -> _
    shift-left: _ -> [w247]
    tunnel: w13 -> [w244]
    tunnel: w12 -> [w243]
    tunnel: w8 -> [w242]
    stop <- w251 stop-if-true
    n87 = call <vilib>:"Parse State Queue__JKI_lib_State_Machine.vi"("State Queue"=w254, "Error In (no error)"=w248) -> ("Remaining States"=w256:string, "Current State"=w241:string, "Arguments"=w255:string)  [unwired: 11 in]
    n88 = feedback #1(w242) -> (w240:string)
    n89 = feedback-in #1(w241) -> ()
    n90 = case shown="\"Action: ClearLogFilePathname\"" w241 {
      selector: w241 -> [w257 _ _ _ _ _ _ _ _ _ _ _ _ _ _ _ _ _ _ _ _ _ _ _]
      tunnel: w256 -> [w264 w274 w525 w537 w549 w554 w560 w589 w612 w615 w622 w630 w633 w653 w658 w661 w673 w694 w698 w723 w789 w799 w817 w820]
      tunnel: w255 -> [_ _ _ _ _ _ _ _ _ _ _ _ _ _ _ _ _ w690 _ w747 w783 w793 _ _]
      tunnel: w249 -> [w265 w272 w523 w534 w547 w557 w559 w567 w595 w614 w619 w626 w632 w639 w657 w660 w666 w692 w705 w733 w784 w794 w813 w819]
      tunnel: [w258 w271 w521 w533 w550 w556 w561 w569 w596 w616 w620 w628 w634 w652 w654 w662 w667 w695 w701 w729 w785 w795 w815 w821] -> w253
      tunnel: w248 -> [_ w270 w520 w532 w551 w556 w561 w571 w603 w616 w620 w628 w634 w649 w654 w662 w669 w695 w702 w737 w786 w796 w809 w821]
      tunnel: [w264 w273 w525 w536 w549 w554 w560 w589 w612 w615 w621 w629 w633 w653 w658 w661 w673 w694 w697 w722 w789 w799 w817 w820] -> w252
      tunnel: [_ _ _ _ _ TRUE _ _ _ _ _ _ _ _ _ _ _ _ _ _ _ _ _ _] -> w251
      tunnel: [w265 w269 w523 w534 w547 w557 w559 w587 w609 w614 w619 w625 w632 w645 w657 w660 w670 w692 w704 w748 w784 w794 w813 w819] -> w250
      tunnel: w247 -> [w263 w268 w524 w535 w548 w553 w558 w588 w611 w613 w618 w627 w631 _ w655 w659 w672 w693 w710 w749 w788 w798 w816 w818]
      tunnel: [w263 w267 w524 w535 w548 w553 w558 w588 w611 w613 w618 w627 w631 w648 w655 w659 w672 w693 w710 w749 w788 w798 w816 w818] -> w246
      tunnel: 100 ("Timeout") -> [_ w266 _ _ _ _ _ _ _ _ _ _ _ _ _ _ _ _ _ _ _ _ _ _]
      tunnel: w240 -> [_ _ _ w531 _ _ _ _ _ _ _ _ _ _ _ _ _ _ _ _ _ _ _ _]
      tunnel: w244 -> [_ _ _ _ _ _ _ _ _ _ w617 _ _ _ _ _ _ _ _ _ _ _ _ _]
      tunnel: w243 -> [_ _ _ _ _ _ _ _ _ _ _ w623 _ _ _ _ _ _ _ _ _ _ _ _]
      frame Default {
        n91 = Format Into String(format string="Software Exception: \nUnhandled State: \"%s\"", w257) -> (resulting string=w261:string)  [unwired: 2 in, 1 out]
        n92 = call <vilib>:"Build Error Cluster_ModKT .vi"("Prepend String (\"\")"=w261, "code"=5001, "error? (F)"=TRUE ("error?")) -> ("error out"=w258:errorcluster)  [unwired: 4 in, 1 out]
      }
      frame "", "EventHandler", "Idle" {
        n93 = event "executes when the state queue is empty" shown="[4] <PublicEvents.LogEngine.AsyncCmd Event>: User Event" {
          selector: w268 -> [_ _ _ _ _ _ _ _ _]
          dyn-events: [_ _ _ _ _ _ _ _ _] -> w267
          timeout: w266 -> [_ _ _ _ _ _ _ _ _]
          tunnel: w274 -> [w276 _ w291 w303 w325 w393 w423 w454 w497]
          tunnel: [w275 w287 w293 w304 w324 w392 w423 w454 w497] -> w273
          tunnel: w272 -> [w277 w289 w294 w297 w322 w389 w416 w447 w488]
          tunnel: [w278 w290 w295 w298 w326 w390 w418 w448 w489] -> w271
          tunnel: w270 -> [w278 w290 w295 w299 w327 w387 w414 w450 w490]
          tunnel: [w277 w288 w294 w296 w321 w391 w415 w451 w491] -> w269
          event Timeout {
            n94 = event-data() -> ()  [unwired: 1 in, 1 out]
            n95 = disable-structure shown="Enabled" {
              disable-tunnel: w276 -> [w280 w285]
              disable-tunnel: [w279 w285] -> w275
              frame Disabled {
                n96 = disable-structure shown="Disabled" {
                  disable-tunnel: ["Loop: Read Data" _] -> w281
                  frame Disabled {
                  }
                  frame Enabled {
                  }
                }
                n97 = call <userlib>:"Periodic Trigger__ogtk.vi"("time (ms)"=u32 1000) -> ("Triggered"=w282:bool)  [unwired: 12 in, 2 out]
                n98 = Select(t=w281, s=w282, f=w280) -> (s? t:f=w279:string)
              }
              frame Enabled {
              }
            }
          }
          event User Event {
            w287 = "Macro: Exit"  # Macro: Exit
            n99 = event-data() -> ("notifier out"=w286:refnum<notifier>)  [unwired: 1 in]
            n100 = Bundle By Name(cluster=w289, "Core.process sync notifier"=w286) -> (w288:T1)
          }
          event "Stop Process": Value Change {
            n101 = event-data() -> ()  [unwired: 1 in, 1 out]
            n102 = call <vilib>:"Add State(s) to Queue__JKI_lib_State_Machine.vi"("State(s) in Front (\"\")"="Macro: Exit", "State(s) in (\"\")"=w291) -> ("States Out"=w293:string)  [unwired: 13 in]
          }
          event "localData": Value Change {
            n103 = event-data() -> ("NewVal"=w302:cluster{"Msg":string, "vData":variant})  [unwired: 1 in]
            n104 = Unbundle(w302) -> ("Msg"=w301:string, "vData"=w300:variant)
            n105 = case shown="\"TDMSLoggerState\"" w301 {
              tunnel: w300 -> [_ w311]
              tunnel: w299 -> [w306 w310]
              tunnel: [w306 w309] -> w298
              tunnel: w297 -> [w305 w308]
              tunnel: [w305 w307] -> w296
              frame "False", Default {
              }
              frame "TDMSLoggerState" {
                n106 = Bundle(FALSE, "Logger State Data"=T7 {"Logger State"=enum."Unknown", "TDMS Logging State"=enum."Unknown", "LogFile path"=path "", "TDMS File path"=path "", "vData"=variant}, path "") -> (w319:cluster{bool, "Logger State Data":T7, path})  [unwired: 1 in]
                n107 = Variant To Data(error in=w310, type=w319, Variant=w311) -> (data=w318:cluster{bool, "Logger State Data":T7, path}, error out=w309:errorcluster)
                n108 = Unbundle(w318) -> (w317:bool, "Logger State Data"=w316:T7, w315:path)
                n109 = Bundle By Name(cluster=w308, "TDMSLogging"=w317, "Logger State Data"=w316, "TDMS file pathname"=w315) -> (w307:T1)
              }
            }
            n110 = call <vilib>:"Add State(s) to Queue__JKI_lib_State_Machine.vi"("State(s) in (\"\")"=w303) -> ("States Out"=w304:string)  [unwired: 14 in]
          }
          event User Event {
            w320 = AsyncCmd_LogEngine--enum."LE.OpenTDMS"  # AsyncMsg
            n111 = event-data() -> ("CmdMsg"=w328:string, "vData"=w329:variant)  [unwired: 1 in, 1 out]
            n112 = call <userlib>:"Set Enum String Value__ogtk.vi"("error in (no error)"=w327, "String Value"=w328, "Default Enum Value"=w320) -> ("error out"=w331:errorcluster, "Enum"=w330:variant)  [unwired: 7 in]
            n113 = Variant To Data(error in=w331, type=w320, Variant=w330) -> (data=w332:T14, error out=w333:errorcluster)
            n114 = case shown="\"LE.ClearLogFilePathname\"" w332 {
              selector: w332 -> [_ _ _ _ w361 w372 _]
              tunnel: w329 -> [_ _ _ w354 _ _ w386]
              tunnel: w333 -> [w338 w342 w345 w353 w362 w373 w385]
              tunnel: [w337 w342 w345 w350 w363 w374 w379] -> w326
              tunnel: ["" "Action: CreateLogFile" "Action: ClearLogFilePathname" w347 w364 w375 _] -> w323
              tunnel: w322 -> [w340 w343 w346 w355 w366 w377 w378]
              tunnel: [w340 w343 w346 w355 w366 w377 w378] -> w321
              frame Default {
                n115 = call <vilib>:"Build Error Cluster_ModKT .vi"("Prepend String (\"\")"="LogEngine Bad Cmd" ("Prepend String (\"\")"), "code"=42, "error? (F)"=TRUE, "error in (no error)"=w338) -> ("error out"=w337:errorcluster)  [unwired: 3 in, 1 out]
              }
              frame "LE.CreateLogFile" {
              }
              frame "LE.ClearLogFilePathname" {
              }
              frame "LE.EnableLogging" {
                n116 = Variant To Data(error in=w353, type=FALSE, Variant=w354) -> (data=w348:bool, error out=w351:errorcluster)
                n117 = Format Into String(format string="Action: EnableLogging >> %s", error in=w351, w348) -> (resulting string=w347:string, error out=w350:errorcluster)  [unwired: 1 in]
              }
              frame "LE.OpenTDMS", "LE.CloseTDMS" {
                w360 = AsyncCmd_LogEngine--enum."LE.OpenTDMS"  # AsyncMsg
                n118 = Equal?(x=w360, y=w361) -> (x = y?=w359:bool)
                n119 = Select(t="Open", s=w359, f="Close") -> (s? t:f=w356:string)
                n120 = Format Into String(format string="Action: OpenCloseTDMS >> %s", error in=w362, w356) -> (resulting string=w364:string, error out=w363:errorcluster)  [unwired: 1 in]
              }
              frame "LE.StartTDMSLogging", "LE.StopTDMSLogging" {
                w371 = AsyncCmd_LogEngine--enum."LE.StartTDMSLogging"  # AsyncMsg
                n121 = Equal?(x=w371, y=w372) -> (x = y?=w370:bool)
                n122 = Select(t="Start", s=w370, f="Stop") -> (s? t:f=w367:string)
                n123 = Format Into String(format string="Action: StartStopTDMS >> %s", error in=w373, w367) -> (resulting string=w375:string, error out=w374:errorcluster)  [unwired: 1 in]
              }
              frame "LE.AppendStrToLog" {
                n124 = Variant To Data(error in=w385, type="", Variant=w386) -> (data=w382:string, error out=w380:errorcluster)
                n125 = Unbundle By Name(w378) -> ("SMQ"=w383:refnum<queue>)
                n126 = call-poly <vilib>:"Polymorphic - Add States(s) To Queue.vi"("queue in"=w383, "state in"="Action: AppendStringToLog", "vData (\"\")"=w382, "error in"=w380) -> ("error out"=w379:errorcluster)  [unwired: 8 in, 3 out]
              }
            }
            n127 = call <vilib>:"Add State(s) to Queue__JKI_lib_State_Machine.vi"("State(s) in Front (\"\")"=w323, "State(s) in (\"\")"=w325) -> ("States Out"=w324:string)  [unwired: 13 in]
          }
          event User Event {
            # "This is not necessary here."
            n128 = event-data() -> ("NEW State Data"=w388:T7)  [unwired: 1 in, 2 out]
            n129 = disable-structure shown="Enabled" {
              disable-tunnel: [w403 w412] -> w391
              disable-tunnel: [w401 w411] -> w390
              disable-tunnel: w389 -> [w398 w412]
              disable-tunnel: w388 -> [w396 _]
              disable-tunnel: w387 -> [w395 w411]
              frame Disabled {
                n130 = Unbundle By Name(w398) -> ("Self Reference"=w397:refnum<class "LogEngine.lvclass">)
                n131 = Unbundle By Name(w396) -> ("Logger State"=w405:T8)
                n132 = disable-structure shown="Enabled" {
                  disable-tunnel: w397 -> [w409 _]
                  disable-tunnel: w396 -> [w408 _]
                  disable-tunnel: w395 -> [w407 w410]
                  disable-tunnel: [w406 w410] -> w394
                  frame Disabled {
                    n133 = property class="LogEngine.lvclass"(reference=w409, error in=w407, "Accessors:Logger State Data*"=w408) -> (error out=w406:errorcluster)  [unwired: 1 out]
                  }
                  frame Enabled {
                  }
                }
                n134 = Equal?(x=w405, y=TD_Logger_State--enum."Logging") -> (x = y?=w400:bool)
                n135 = Bundle By Name(cluster=w398, "Logging"=w400) -> (w403:T1)
                n136 = Unbundle By Name(w403) -> ("SMQ"=w402:refnum<queue>)
                n137 = call <vilib>:"Add State to Queue with vData.vi"("queue in"=w402, "state in"="Action: UpdateSMData >> LoggerState", "vData (\"\")"=w400, "error in"=w394) -> ("error out"=w401:errorcluster)  [unwired: 8 in, 3 out]
              }
              frame Enabled {
              }
            }
            n138 = call <vilib>:"Add State(s) to Queue__JKI_lib_State_Machine.vi"("State(s) in (\"\")"=w393) -> ("States Out"=w392:string)  [unwired: 14 in]
          }
          event User Event {
            n139 = event-data() -> ("CmdMsg"=w422:string, "vData"=w419:variant)  [unwired: 1 in, 1 out]
            n140 = Unbundle By Name(w416) -> ("Self Reference"=w420:refnum<class "LogEngine.lvclass">)
            n141 = Unbundle By Name(w416) -> ("SMQ"=w417:refnum<queue>)
            n142 = call "get async msg.vi"("error in (no error)"=w414, "Msg String in"=w422) -> ("error out"=w413:errorcluster, "AsyncMsg"=w421:T15)  [unwired: 8 in]
            n143 = case shown="\"Application.SendSessionSettings\"" w421 {
              tunnel: w420 -> [_ _ w441]
              tunnel: w419 -> [_ _ w442]
              tunnel: w413 -> [w425 w427 w435]
              tunnel: [w425 w427 w432] -> w418
              tunnel: w417 -> [_ _ w431]
              tunnel: w416 -> [_ _ _]
              tunnel: w416 -> [w424 w426 w430]
              tunnel: [w424 w426 w429] -> w415
              frame "Application.AppClassReference", Default {
              }
              frame "Application.RefreshSettings" {
              }
              frame "Application.SendSessionSettings" {
                n144 = Variant To Data(error in=w435, type=T5 {"Job_ID"="", "Operator_ID"="", "Station_ID"="", "Job_Description"=""} ("Session Settings"), Variant=w442) -> (data=w428:T5, error out=w440:errorcluster)
                n145 = call "Get ObjData.vi"("error in (no error)"=w440, "LogEngine"=w441) -> ("error out"=w436:errorcluster, "Obj Data"=w438:T16, "LogEngine out"=w439:refnum<class "LogEngine.lvclass">)  [unwired: 7 in]
                n146 = Bundle By Name(cluster=w438, "LogHeaderData.SessionSettings"=w428) -> (w437:T16)
                n147 = call "Set ObjData.vi"("error in (no error)"=w436, "Obj Data"=w437, "LogEngine"=w439) -> ("error out"=w433:errorcluster)  [unwired: 7 in, 1 out]
                n148 = Bundle By Name(cluster=w430, "LogHeaderData.SessionSettings"=w428) -> (w429:T1)
                n149 = call <vilib>:"Add State to Queue with vData.vi"("queue in"=w431, "state in"="Action: UpdateSMData >> SessionSettings", "vData (\"\")"=w428, "error in"=w433) -> ("error out"=w432:errorcluster)  [unwired: 8 in, 3 out]
              }
            }
          }
          event User Event {
            n150 = event-data() -> ("CmdMsg"=w444:string, "vData"=w445:variant)  [unwired: 1 in, 1 out]
            n151 = Unbundle By Name(w447) -> ("Self Reference"=w446:refnum<class "LogEngine.lvclass">)
            n152 = Unbundle By Name(w447) -> ("Sequencer"=w452:refnum<class "Sequencer.lvclass">)
            n153 = call "get async msg.vi"("error in (no error)"=w450, "Msg String in"=w444) -> ("error out"=w449:errorcluster, "AsyncMsg"=w453:T17)  [unwired: 8 in]
            n154 = case shown="\"Sequencer.LoadSeqStatusChg\"" w453 {
              tunnel: w445 -> [_ w464 _]
              tunnel: w452 -> [_ w467 _]
              tunnel: w449 -> [w456 w463 w485]
              tunnel: w447 -> [_ _ w486]
              tunnel: [w455 w466 w486] -> w451
              tunnel: w447 -> [w455 w465 _]
              tunnel: [w456 w461 w485] -> w448
              tunnel: w446 -> [_ w460 _]
              frame "Sequencer.SeqStepChg" {
              }
              frame "Sequencer.LoadSeqStatusChg" {
                (unwired) LoadSeqStatus--enum."Unknown" ("LoadSeqStatus")
                n155 = Variant To Data(error in=w463, type=T11 {"Time Stamp"=timestamp(0 s since 1904-01-01), "OLD Status"=enum."Unknown", "NEW Status"=enum."Unknown"} ("LoadSeqStatus EvData"), Variant=w464) -> (data=w458:T11, error out=w462:errorcluster)
                n156 = Unbundle(w458) -> ("NEW Status"=w457:T12)  [unwired: 2 out]
                n157 = case shown="\"Loaded\"" w457 {
                  tunnel: w467 -> [_ w484]
                  tunnel: [w468 w482] -> w466
                  tunnel: w465 -> [w468 w480]
                  tunnel: w462 -> [w469 w479]
                  tunnel: [w469 w472] -> w461
                  tunnel: w460 -> [_ w474]
                  frame "Unknown", Default {
                  }
                  frame "Loaded" {
                    n158 = property class="Sequencer.lvclass"(reference=w484, error in=w479) -> (error out=w473:errorcluster, "Accessors:SeqData*"=w483, "Accessors:SeqFile*"=w481)  [unwired: 1 out]
                    n159 = Unbundle By Name(w483) -> ("SeqFileParams"=w471)
                    n160 = Path To String(path=w481) -> (string=w470:string)
                    n161 = call "Get ObjData.vi"("error in (no error)"=w473, "LogEngine"=w474) -> ("error out"=w475:errorcluster, "Obj Data"=w477:T16, "LogEngine out"=w478:refnum<class "LogEngine.lvclass">)  [unwired: 7 in]
                    n162 = Bundle By Name(cluster=w477, "SeqFileParams"=w471, "LogHeaderData.SequenceFile"=w470) -> (w476:T16)
                    n163 = Bundle By Name(cluster=w480, "SeqFileParams"=w471, "LogHeaderData.SequenceFile"=w470) -> (w482:T1)
                    n164 = call "Set ObjData.vi"("error in (no error)"=w475, "Obj Data"=w476, "LogEngine"=w478) -> ("error out"=w472:errorcluster)  [unwired: 7 in, 1 out]
                  }
                }
              }
              frame "Sequencer.SeqExecStatusChg" {
                # "Potentially use this event to start logging."
              }
            }
          }
          event User Event {
            n165 = event-data() -> ("CmdMsg"=w496:string, "vData"=w493:variant)  [unwired: 1 in, 1 out]
            n166 = Unbundle By Name(w488) -> ("Self Reference"=w487:refnum<class "LogEngine.lvclass">)
            n167 = Scan From String(input string=w496, error in=w490, default 1=AsyncMsg_DAQ--enum."DAQ.SendAI_InstSettings" ("AsyncMsg")) -> (error out=w492:errorcluster, output 1=w494:T13)  [unwired: 2 in, 2 out]
            n168 = case shown="\"DAQ.SendAI_InstSettings\"" w494 {
              tunnel: w493 -> [_ w518]
              tunnel: w492 -> [w498 w517]
              tunnel: w488 -> [w499 w515]
              tunnel: [w499 w511] -> w491
              tunnel: [w498 w505] -> w489
              tunnel: w487 -> [_ w502]
              frame Default {
              }
              frame "DAQ.SendAI_InstSettings" {
                w513 = ""  # AI TaskName
                w514 = T18 {"DaqRate"=0.0, "NumSamples"=0}  # AI InstSettings
                n169 = Bundle("AI InstSettings"=w514, "AI TaskName"=w513) -> (w516:T19)  [unwired: 1 in]
                n170 = Variant To Data(error in=w517, type=w516, Variant=w518) -> (data=w512:T19, error out=w506:errorcluster)
                n171 = Unbundle By Name(w512) -> ("AI InstSettings.DaqRate"=w500:dbl, "AI InstSettings.NumSamples"=w503:i32, "AI TaskName"=w504:string)
                n172 = call "Get ObjData.vi"("error in (no error)"=w506, "LogEngine"=w502) -> ("error out"=w507:errorcluster, "Obj Data"=w509:T16, "LogEngine out"=w510:refnum<class "LogEngine.lvclass">)  [unwired: 7 in]
                n173 = Reciprocal(x=w500) -> (1/x=w501:dbl)
                n174 = Bundle By Name(cluster=w509, "LogHeaderData.SamplingRate"=w500, "LogHeaderData.SamplesPerAcq"=w503, "LogHeaderData.AI TaskName"=w504) -> (w508:T16)
                n175 = Bundle By Name(cluster=w515, "dt(s)"=w501, "LogHeaderData.SamplingRate"=w500, "LogHeaderData.SamplesPerAcq"=w503, "LogHeaderData.AI TaskName"=w504) -> (w511:T1)
                n176 = call "Set ObjData.vi"("error in (no error)"=w507, "Obj Data"=w508, "LogEngine"=w510) -> ("error out"=w505:errorcluster)  [unwired: 7 in, 1 out]
              }
            }
          }
        }
      }
      frame "Process Sync" {
        n177 = Unbundle By Name(w523) -> ("Core.process sync notifier"=w522:refnum<notifier>, "quitting"=w519:bool)
        n178 = case shown="False" w519 {
          tunnel: w522 -> [w529 _]
          tunnel: [w528 w530] -> w521
          tunnel: w520 -> [w526 w530]
          frame False {
            n179 = Send Notification(notification=TRUE, notifier=w529, error in (no error)=w526) -> (error out=w528:errorcluster)  [unwired: 1 out]
          }
          frame True {
          }
        }
      }
      frame "Error Handler" {
        n180 = disable-structure shown="Enabled" {
          disable-tunnel: [w540 errorcluster {"status"=FALSE, "code"=0, "source"=""} ("error constant")] -> w533
          disable-tunnel: w532 -> [w539 w543]
          disable-tunnel: w531 -> [w538 _]
          frame Enabled {
            n181 = Concatenate Strings("Event Handler Loop\nPrevious State: ", w538) -> (w541:string)
            n182 = call "Handle Error SM.vi"("error in (no error)"=w539, "CustomMessage"=w541) -> ("error out"=w540:errorcluster)  [unwired: 7 in, 2 out]
          }
          frame Disabled {
            n183 = call <vilib>:"General Error Handler.vi"("error in (no error)"=w543) -> ()  [unwired: 10 in, 5 out]
          }
        }
        n184 = call <vilib>:"Add State(s) to Queue__JKI_lib_State_Machine.vi"("State(s) in (\"\")"=w537) -> ("States Out"=w536:string)  [unwired: 14 in]
      }
      frame "CleanUp" {
        n185 = Unbundle By Name(w547) -> ("Self Reference"=w546:refnum<class "LogEngine.lvclass">)
        n186 = Unbundle By Name(w547) -> ("Core.Current VI Ref"=w552:refnum<vi>)
        n187 = Close Reference(reference=w552, error in (no error)=w551) -> (error out=w550:errorcluster)
        n188 = call "Fire LogEngineStateChanged Event_LogEngine.vi"("NEW State Data"=T7 {"Logger State"=enum."Unknown", "TDMS Logging State"=enum."Unknown", "LogFile path"=path "", "TDMS File path"=path "", "vData"=variant}, "LogEngine"=w546) -> ()  [unwired: 8 in, 2 out]
      }
      frame "Exit" {
      }
      frame "------ Data ------" {
      }
      frame "Data: Initialize2" {
        w568 = "Action: UpdateSMData >> Log&TDMS_Folders"
        n189 = Unbundle By Name(w567) -> ("Self Reference"=w573:refnum<class "LogEngine.lvclass">)
        n190 = Unbundle By Name(w567) -> ("SMQ"=w566:refnum<queue>, "TDMS SMQ"=w565:refnum<queue>)
        n191 = call "FG - FilePathnames.vi"() -> ("FilePaths out"=w572:T10)  [unwired: 4 in, 1 out]
        n192 = property class="LogEngine.lvclass"(reference=w573) -> ("Accessors:Settings*"=w574:T6)  [unwired: 1 in, 2 out]
        n193 = Unbundle By Name(w572) -> ("DataLogFolder"=w579:path)
        n194 = Unbundle By Name(w574) -> ("LogFile folder name"=w576:string, "TDMS folder name"=w578:string)
        n195 = Build Path(base path=w579, name or relative path=w578) -> (appended path=w577:path)
        n196 = Build Path(base path=w579, name or relative path=w576) -> (appended path=w575:path)
        n197 = call <userlib>:"Create Dir if Non-Existant__ogtk.vi"("Directory Path"=w577) -> ("dup Directory Path"=w564:path)  [unwired: 8 in, 2 out]
        n198 = call <userlib>:"Create Dir if Non-Existant__ogtk.vi"("Directory Path"=w575) -> ("dup Directory Path"=w563:path)  [unwired: 8 in, 2 out]
        n199 = Bundle("dup Directory Path"=w563, "dup Directory Path"=w564) -> (w562:T20)  [unwired: 1 in]
        n200 = Bundle By Name(cluster=w567, "LogFile pathname"=path "", "HeaderStr Created?"=FALSE, "TDMSLogging"=FALSE, "Logging"=FALSE, "tdms fileref"=refnum<k0> refnum, "Logger State Data"=T7 {"Logger State"=enum."Unknown", "TDMS Logging State"=enum."Unknown", "LogFile path"=path "", "TDMS File path"=path "", "vData"=variant}, "TDMS file pathname"=path "", "LogFile folder"=w563, "TDMS folder"=w564) -> (w587:T1)
        n201 = call <vilib>:"Add State to Queue with vData.vi"("queue in"=w565, "state in"=w568, "vData (\"\")"=w562, "error in"=w571) -> ("error out"=w570:errorcluster)  [unwired: 8 in, 3 out]
        n202 = call <vilib>:"Add State to Queue with vData.vi"("queue in"=w566, "state in"=w568, "vData (\"\")"=w562, "error in"=w570) -> ("error out"=w569:errorcluster)  [unwired: 8 in, 3 out]
      }
      frame "Data: Initialize" {
        # "#NOTE: KT 2019-0713\nPresently, AVC2 application\nhas only one AI task, and therefore\nonly one set of AI Settings"
        n203 = Unbundle By Name(w595) -> ("Self Reference"=w594:refnum<class "LogEngine.lvclass">)
        n204 = Unbundle By Name(w595) -> ("DAQ"=w606:refnum<class "DAQ.lvclass">)
        n205 = property class="DAQ"(reference=w606, error in=w603) -> (error out=w597:errorcluster, "Accessors:AI Settings*"=w605:T21[])  [unwired: 1 out]
        n206 = Index Array(array=w605, index=0) -> (element=w604:T21)
        n207 = Unbundle By Name(w604) -> ("AI TaskName"=w593:string, "AI InstSettings.DaqRate"=w590:dbl, "AI InstSettings.NumSamples"=w592:i32)
        n208 = control-ref of="Current VI Reference"() -> (w610:refnum<vi>)
        n209 = Reciprocal(x=w590) -> (1/x=w591:dbl)
        n210 = call "Get ObjData.vi"("error in (no error)"=w597, "LogEngine"=w594) -> ("error out"=w598:errorcluster, "Obj Data"=w600:T16, "LogEngine out"=w601:refnum<class "LogEngine.lvclass">)  [unwired: 7 in]
        n211 = Bundle By Name(cluster=w600, "LogHeaderData.AI TaskName"=w593, "LogHeaderData.SamplingRate"=w590, "LogHeaderData.SamplesPerAcq"=w592) -> (w599:T16)
        n212 = Bundle By Name(cluster=w595, "Core.Current VI Ref"=w610, "Core.process sync notifier"="start process sync notifier", "quitting"=FALSE, "LogHeaderData.AI TaskName"=w593, "LogHeaderData.SamplingRate"=w590, "LogHeaderData.SamplesPerAcq"=w592, "dt(s)"=w591) -> (w609:T1)
        n213 = call "Set ObjData.vi"("error in (no error)"=w598, "Obj Data"=w599, "LogEngine"=w601) -> ("error out"=w596:errorcluster)  [unwired: 7 in, 1 out]
      }
      frame "------ Macro ------" {
      }
      frame "Macro: Initialize" {
        n214 = call <vilib>:"Add State(s) to Queue__JKI_lib_State_Machine.vi"("State(s) in Front (\"\")"=w617, "State(s) in (\"\")"=w622) -> ("States Out"=w621:string)  [unwired: 13 in]
      }
      frame "Macro: Exit" {
        n215 = Bundle By Name(cluster=w626, "quitting"=TRUE) -> (w625:T1)
        n216 = call <vilib>:"Add State(s) to Queue__JKI_lib_State_Machine.vi"("State(s) in Front (\"\")"=w623, "State(s) in (\"\")"=w630) -> ("States Out"=w629:string)  [unwired: 13 in]
      }
      frame "------ UI ------" {
      }
      frame "UI: Register Events" {
        n217 = Unbundle By Name(w639) -> ("Self Reference"=w650:refnum<class "LogEngine.lvclass">)
        n218 = Unbundle By Name(w639) -> ("Sequencer"=w643:refnum<class "Sequencer.lvclass">)
        n219 = Unbundle By Name(w639) -> ("DAQ"=w638:refnum<class "DAQ.lvclass">)
        n220 = call "Get Public Events.vi"("error in (no error)"=w649, "LogEngine.lvclass"=w650) -> ("error out"=w640:errorcluster, "PublicEvents"=w651:T23)  [unwired: 7 in, 1 out]
        n221 = call "FG - App Class Ref.vi"() -> ("Application out"=w647:refnum<class "Application.lvclass">)  [unwired: 9 in, 1 out]
        n222 = call "Get PublicEvents.vi"("error in (no error)"=w640, "Application in"=w647) -> ("error out"=w642:errorcluster, "Public Events"=w646:T24, "Application out"=w644:refnum<class "Application.lvclass">)  [unwired: 7 in]
        n223 = call "Get PublicEvents.vi"("error in (no error)"=w642, "Sequencer in"=w643) -> ("error out"=w637:errorcluster, "Public Events"=w641:T25)  [unwired: 7 in, 1 out]
        n224 = call "Get Public Events.vi"("error in (no error)"=w637, "DAQ"=w638) -> ("error out"=w636:errorcluster, "PublicEvents"=w635:T26)  [unwired: 7 in, 1 out]
        n225 = Bundle By Name(cluster=w639, "Application"=w644) -> (w645:T1)
        n226 = register-events(error in=w636, w651, w646, w641, w635) -> (reference out=w648:refnum<event-registration>, error out=w652:errorcluster)  [unwired: 1 in]
      }
      frame "UI: Unregister Events" {
        n227 = Unregister For Events(event registration refnum=w655, error in=w654) -> (error out=w656:errorcluster)
        n228 = call <vilib>:"Clear Errors.vi"("error in (no error)"=w656) -> ()  [unwired: 5 in, 2 out]
      }
      frame "------ Action ------" {
      }
      frame "Action: ClearLogFilePathname" {
        n229 = Unbundle By Name(w666) -> ("Logging"=w663:bool, "Self Reference"=w671:refnum<class "LogEngine.lvclass">)
        n230 = Unbundle By Name(w666) -> ("SMQ"=w665:refnum<queue>)
        n231 = case shown="False" w663 {
          tunnel: w671 -> [w683 _]
          tunnel: [w679 w688] -> w670
          tunnel: w669 -> [w677 w686]
          tunnel: [w676 w685] -> w668
          tunnel: w666 -> [w675 w688]
          frame False {
            w678 = path ""
            n232 = call "Get Logger State Data.vi"("error in (no error)"=w677, "LogEngine"=w683) -> ("error out"=w682:errorcluster, "Logger State Data"=w674:T7, "LogEngine out"=w681:refnum<class "LogEngine.lvclass">)  [unwired: 7 in]
            n233 = Bundle By Name(cluster=w674, "LogFile path"=w678) -> (w680:T7)
            n234 = call "Fire LogEngineStateChanged Event_LogEngine.vi"("error in (no error)"=w682, "NEW State Data"=w680, "LogEngine"=w681) -> ("error out"=w676:errorcluster)  [unwired: 7 in, 1 out]
            n235 = Bundle By Name(cluster=w675, "LogFile pathname"=w678) -> (w679:T1)
          }
          frame True {
            n236 = call "Dialog Box Timeout v2.vi"("Error In"=w686, "Timeout (s)"=4.0, "Message"="Logging is enabled.\nCannot clear log file pathname") -> ("Error Out"=w685:errorcluster)  [unwired: 8 in]
          }
        }
        n237 = call <vilib>:"Add State to Queue with vData.vi"("queue in"=w665, "state in"="Action: UpdateSMData >> ClearLogFilePathname", "bypass (F)"=w663, "error in"=w668) -> ("error out"=w667:errorcluster)  [unwired: 8 in, 3 out]
      }
      frame "Action: SendStatusMsg" {
        n238 = Unbundle By Name(w692) -> ("StatusStr Ref"=w691:refnum<vi>)
        n239 = call <vilib>:"format status message v2.vi"("status msg"=w690, "Str Refnum"=w691) -> ("error out"=w689:errorcluster)  [unwired: 5 in, 4 out]
        n240 = call <userlib>:"Clear All Errors__ogtk.vi"("Error In"=w689) -> ()  [unwired: 3 in, 1 out]
      }
      frame "Action: CreateLogFile" {
        n241 = Unbundle By Name(w705) -> ("LogFile folder"=w706:path, "Self Reference"=w707:refnum<class "LogEngine.lvclass">)
        n242 = call "Create Log Header String.vi"("error in (no error)"=w702, "LogEngine in"=w707) -> ("error out"=w708:errorcluster, "LogHeaderString"=w709:string)  [unwired: 7 in, 1 out]
        n243 = call "Create Log File.vi"("error in (no error)"=w708, "LogHeader String"=w709, "LogFile Folder"=w706) -> ("error out"=w701:errorcluster, "new file path"=w703:path)  [unwired: 7 in]
        n244 = case shown="No Error" w701 {
          tunnel: w705 -> [w715 w720]
          tunnel: [w714 w719] -> w704
          tunnel: w703 -> [w713 _]
          tunnel: ["LogFile Created" "LogFile NOT Created"] -> w699
          frame No Error {
            n245 = Bundle By Name(cluster=w715, "LogFile pathname"=w713, "HeaderStr Created?"=TRUE) -> (w714:T1)
          }
          frame Error {
            n246 = Bundle By Name(cluster=w720, "LogFile pathname"=path "", "HeaderStr Created?"=FALSE) -> (w719:T1)
          }
        }
        n247 = Format Into String(format string="Action: SendStatusMsg >> %s", w699) -> (resulting string=w696:string)  [unwired: 2 in, 1 out]
        n248 = call <vilib>:"Add State(s) to Queue__JKI_lib_State_Machine.vi"("State(s) in Front (\"\")"=w696, "State(s) in (\"\")"=w698) -> ("States Out"=w697:string)  [unwired: 13 in]
      }
      frame "Action: EnableLogging" {
        w726 = "Action: UpdateSMData >> LoggerState"
        n249 = Unbundle By Name(w733) -> ("LogFile pathname"=w743:path, "HeaderStr Created?"=w740:bool)
        n250 = Unbundle By Name(w733) -> ("Self Reference"=w746:refnum<class "LogEngine.lvclass">)
        n251 = Unbundle By Name(w733) -> ("TDMS SMQ"=w728:refnum<queue>, "SMQ"=w732:refnum<queue>)
        n252 = call "Get Logger State Data.vi"("error in (no error)"=w737, "LogEngine"=w746) -> ("error out"=w738:errorcluster, "Logger State Data"=w744:T7, "LogEngine out"=w745:refnum<class "LogEngine.lvclass">)  [unwired: 7 in]
        n253 = case shown="\"False\", Default" w747 {
          tunnel: w745 -> [w757 w765]
          tunnel: w744 -> [w755 w767]
          tunnel: w743 -> [w750 w766]
          tunnel: [w757 w765] -> w742
          tunnel: [w752 w764] -> w741
          tunnel: [w752 w762] -> w734
          tunnel: w740 -> [_ w761]
          tunnel: [FALSE ("HeaderStr Created?") w760] -> w739
          tunnel: [FALSE w763] -> w735
          tunnel: [w750 w759] -> w731
          tunnel: ["Logging Disabled" w758] -> w724
          frame "False", Default {
            n254 = Bundle By Name(cluster=w755, "Logger State"=TD_Logger_State--enum."NotLogging") -> (w752:T7)
          }
          frame "True" {
            n255 = case shown="False" w761 {
              selector: w761 -> [_ w777]
              tunnel: w767 -> [w774 w781]
              tunnel: w766 -> [w769 w776]
              tunnel: [w774 w778] -> w764
              tunnel: [FALSE TRUE] -> w763
              tunnel: [w774 w778] -> w762
              tunnel: [FALSE w777] -> w760
              tunnel: [w769 w776] -> w759
              tunnel: ["Logging Disabled" "Logging Enabled"] -> w758
              frame False {
                n256 = call "Dialog Box Timeout v2.vi"("Timeout (s)"=5.0, "Message"="Logfile Header Must Be Created Before Logging Is Enabled.") -> ()  [unwired: 9 in, 1 out]
              }
              frame True {
                n257 = Bundle By Name(cluster=w781, "Logger State"=TD_Logger_State--enum."Logging", "LogFile path"=w776) -> (w778:T7)
              }
            }
          }
        }
        n258 = Format Into String(format string="Action: SendStatusMsg >> %s", w724) -> (resulting string=w721:string)  [unwired: 2 in, 1 out]
        n259 = call "Fire LogEngineStateChanged Event_LogEngine.vi"("error in (no error)"=w738, "NEW State Data"=w741, "LogEngine"=w742) -> ("error out"=w736:errorcluster)  [unwired: 7 in, 1 out]
        n260 = Bundle(w735, "Logger State Data"=w734, "LogFile pathname"=w731) -> (w727:T27)  [unwired: 1 in]
        n261 = Bundle By Name(cluster=w733, "Logger State Data"=w734, "Logging"=w735, "HeaderStr Created?"=w739, "LogFile pathname"=w731) -> (w748:T1)
        n262 = call <vilib>:"Add State(s) to Queue__JKI_lib_State_Machine.vi"("State(s) in Front (\"\")"=w721, "State(s) in (\"\")"=w723) -> ("States Out"=w722:string)  [unwired: 13 in]
        n263 = call <vilib>:"Add State to Queue with vData.vi"("queue in"=w732, "state in"=w726, "vData (\"\")"=w727, "error in"=w736) -> ("error out"=w730:errorcluster)  [unwired: 8 in, 3 out]
        n264 = call <vilib>:"Add State to Queue with vData.vi"("queue in"=w728, "state in"=w726, "vData (\"\")"=w727, "error in"=w730) -> ("error out"=w729:errorcluster)  [unwired: 8 in, 3 out]
      }
      frame "Action: OpenCloseTDMS" {
        n265 = case shown="\"Close\"" w783 {
          tunnel: [_ "CMD: CloseTDMSFileRef" "CMD: OpenTDMSFileRef"] -> w782
          frame Default {
          }
          frame "Close" {
          }
          frame "Open" {
          }
        }
        n266 = Unbundle By Name(w784) -> ("TDMS SMQ"=w787:refnum<queue>)
        n267 = call <vilib>:"Add State to Queue with vData.vi"("queue in"=w787, "state in"=w782, "error in"=w786) -> ("error out"=w785:errorcluster)  [unwired: 9 in, 3 out]
      }
      frame "Action: StartStopTDMS" {
        n268 = case shown="\"Stop\"" w793 {
          tunnel: [_ "CMD: StopTDMSLogging" "CMD: StartTDMSLogging"] -> w792
          frame Default {
          }
          frame "Stop" {
          }
          frame "Start" {
          }
        }
        n269 = Unbundle By Name(w794) -> ("TDMS SMQ"=w797:refnum<queue>)
        n270 = call <vilib>:"Add State to Queue with vData.vi"("queue in"=w797, "state in"=w792, "error in"=w796) -> ("error out"=w795:errorcluster)  [unwired: 9 in, 3 out]
      }
      frame "Action: TerminateAsyncThreads" {
        n271 = Unbundle By Name(w813) -> ("TDMS SMQ"=w802:refnum<queue>, "SMQ"=w812:refnum<queue>)
        n272 = Flush Queue(queue=w812) -> (queue out=w808:refnum<queue>)  [unwired: 1 in, 2 out]
        n273 = call <vilib>:"Add State to Queue with vData.vi"("queue in"=w808, "mode (back)"=enum16{"back", "front"}."front", "state in"="Macro: Exit", "error in"=w809) -> ("error out"=w804:errorcluster)  [unwired: 8 in, 3 out]
        n274 = Flush Queue(queue=w802) -> (queue out=w807:refnum<queue>)  [unwired: 1 in, 2 out]
        n275 = call <vilib>:"Add State to Queue with vData.vi"("queue in"=w807, "mode (back)"=enum16{"back", "front"}."front", "state in"="Macro: Exit", "error in"=w804) -> ("error out"=w803:errorcluster)  [unwired: 8 in, 3 out]
        n276 = call <userlib>:"Wait (ms)__ogtk.vi"("error in (no error)"=w803, "milliseconds to wait"=u32 1000) -> ("error out"=w815:errorcluster)  [unwired: 8 in, 1 out]
      }
      frame "Loop: Read Data" {
        # "No Op ??"
      }
    }
  }
  n277 = while {
    shift-right: [w823] -> _
    shift-left: w6 -> [w824]
    tunnel: w5 -> [w834]
    shift-right: [w826] -> w4
    shift-left: w7 -> [w828]
    stop <- w825 stop-if-true
    # "TDMS Async Logging Loop"
    n278 = call <vilib>:"Get Next Queued State with vData.vi"("queue in"=w834, "error in (no error)"=w828, "timeout (100)"=40) -> ("vData out"=w829:variant, "queue out"=w832:refnum<queue>, "Next State"=w833:string, "queued msg"=w831:string, "Prev State"=w830:string, "error out"=w827:errorcluster)  [unwired: 6 in, 1 out]
    n279 = case shown="\"Action: SendStatusMsg\"" w833 {
      tunnel: w827 -> [_ w843 w854 _ w881 w896 w911 w916 w918 w926 w940 w981 w1029 w1035 w1040 w1042 w1090 w1103 w1109 w1110]
      tunnel: w832 -> [_ _ _ w880 w882 w897 _ w913 _ w919 w932 w967 w1010 _ _ _ _ _ _ _]
      tunnel: w831 -> [_ _ _ _ _ _ _ _ _ _ _ _ _ _ w1036 w1045 _ _ _ _]
      selector: w833 -> [w835 _ _ _ _ _ _ _ _ _ _ _ _ _ _ _ _ _ _ _]
      tunnel: w830 -> [_ w842 _ _ _ _ _ _ _ _ _ _ _ _ _ _ _ _ _ _]
      tunnel: w829 -> [_ _ _ _ _ _ _ _ _ _ _ _ _ _ _ w1046 _ _ _ w1113]
      tunnel: [w836 w844 w854 w875 w881 w895 w911 w914 w918 w920 w933 w972 w1011 w1035 w1040 w1041 w1089 w1101 w1109 w1114] -> w826
      tunnel: [_ _ _ _ TRUE _ _ _ _ _ _ _ _ _ _ _ _ _ _ _] -> w825
      tunnel: w824 -> [w841 w845 w853 w874 w883 w898 w910 w915 w917 w929 w937 w980 w1014 w1034 w1037 w1044 w1080 w1099 w1108 w1112]
      tunnel: [w841 w845 w855 w873 w883 w898 w910 w915 w917 w925 w938 w987 w1030 w1034 w1037 w1043 w1080 w1099 w1108 w1111] -> w823
      frame Default {
        n280 = Format Into String(format string="Software Exception: \nUnhandled State: \"%s\"", w835) -> (resulting string=w838:string)  [unwired: 2 in, 1 out]
        n281 = call <vilib>:"Build Error Cluster_ModKT .vi"("Prepend String (\"\")"=w838, "code"=5001, "error? (F)"=TRUE ("error?")) -> ("error out"=w836:errorcluster)  [unwired: 4 in, 1 out]
      }
      frame "Error Handler" {
        n282 = disable-structure shown="Enabled" {
          disable-tunnel: [w848 errorcluster {"status"=FALSE, "code"=0, "source"=""} ("error constant")] -> w844
          disable-tunnel: w843 -> [w847 w851]
          disable-tunnel: w842 -> [w846 _]
          frame Enabled {
            n283 = Concatenate Strings("TDMS Loggnig Loop\nPrevious State: ", w846) -> (w849:string)
            n284 = call "Handle Error SM.vi"("error in (no error)"=w847, "CustomMessage"=w849) -> ("error out"=w848:errorcluster)  [unwired: 7 in, 2 out]
          }
          frame Disabled {
            n285 = call <vilib>:"General Error Handler.vi"("error in (no error)"=w851) -> ()  [unwired: 10 in, 5 out]
          }
        }
      }
      frame "Initialize" {
        n286 = disable-structure shown="Enabled" {
          disable-tunnel: [w869 w870] -> w855
          disable-tunnel: w853 -> [w865 w870]
          frame Disabled {
            n287 = Unbundle By Name(w865) -> ("Self Reference"=w864:refnum<class "LogEngine.lvclass">)
            n288 = call "FG - FilePathnames.vi"() -> ("FilePaths out"=w866:T10)  [unwired: 4 in, 1 out]
            n289 = property class="LogEngine.lvclass"(reference=w864) -> ("Accessors:Settings*"=w863:T6)  [unwired: 1 in, 2 out]
            n290 = Unbundle By Name(w866) -> ("DataLogFolder"=w858:path)
            n291 = Unbundle By Name(w863) -> ("LogFile folder name"=w861:string, "TDMS folder name"=w859:string)
            n292 = Build Path(base path=w858, name or relative path=w859) -> (appended path=w860:path)
            n293 = Build Path(base path=w858, name or relative path=w861) -> (appended path=w862:path)
            n294 = call <userlib>:"Create Dir if Non-Existant__ogtk.vi"("Directory Path"=w860) -> ("dup Directory Path"=w856:path)  [unwired: 8 in, 2 out]
            n295 = call <userlib>:"Create Dir if Non-Existant__ogtk.vi"("Directory Path"=w862) -> ("dup Directory Path"=w857:path)  [unwired: 8 in, 2 out]
            n296 = Bundle By Name(cluster=w865, "Logging"=FALSE, "tdms fileref"=refnum<k0> refnum, "LogFile folder"=w857, "TDMS folder"=w856) -> (w869:T1)
          }
          frame Enabled {
          }
        }
      }
      frame "CleanUp", "Macro: Exit" {
        # "Do any necessary async loop clean up here before quitting"
        n297 = Flush Queue(queue=w880, error in (no error)=errorcluster {"status"=FALSE, "code"=0, "source"=""}) -> (queue out=w876:refnum<queue>, error out=w878:errorcluster)  [unwired: 1 out]
        n298 = call-poly <vilib>:"Polymorphic - Add States(s) To Queue.vi"("queue in"=w876, "states in"="CMD: StopTDMSLogging\nCMD: CloseTDMSFileRef\nExit", "error in"=w878) -> ("error out"=w875:errorcluster)  [unwired: 10 in, 2 out]
        n299 = Bundle By Name(cluster=w874, "quitting"=TRUE, "TDMSLogging"=FALSE) -> (w873:T1)
      }
      frame "Exit" {
        n300 = disable-structure shown="Disabled" {
          disable-tunnel: w882 -> [w885 _]
          frame Disabled {
            n301 = Release Queue(queue=w885, force destroy? (F)=TRUE) -> ()  [unwired: 1 in, 3 out]
          }
          frame Enabled {
          }
        }
      }
      frame "", "Idle" {
        # "ExecTDMSLogData needs to execute continuously\neven if Logging is not enabled because\nit will flush the queue if not being dequeued\nfor writing."
        n302 = Unbundle By Name(w898) -> ("LogEngine Settings.LogWriteIntv (ms)"=w889:u32)  [unwired: 1 out]
        n303 = In Range and Coerce(upper limit=u32 30000, x=w889, lower limit=u32 50) -> (coerced(x)=w890:u32)  [unwired: 1 out]
        n304 = First Call?() -> (First Call?: T/F=w894:bool)
        n305 = call <userlib>:"Periodic Trigger__ogtk.vi"("time (ms)"=w890, "reset"=w894) -> ("Triggered"=w893:bool)  [unwired: 11 in, 2 out]
        n306 = Compound Arithmetic op=AND(w893, TRUE ("value")) -> (w892:bool)
        n307 = case shown="True" w892 {
          tunnel: w897 -> [w900 w909]
          tunnel: w896 -> [w904 w907]
          tunnel: [w901 w906] -> w895
          frame False {
            w899 = TRUE  # bypass (F)
            n308 = call <userlib>:"Wait (ms)__ogtk.vi"("error in (no error)"=w904, "milliseconds to wait"=u32 100) -> ("error out"=w902:errorcluster)  [unwired: 8 in, 1 out]
            n309 = call <vilib>:"Add State to Queue with vData.vi"("queue in"=w900, "state in"="Action: FlushRawDataQ", "bypass (F)"=w899, "error in"=w902) -> ("error out"=w901:errorcluster)  [unwired: 8 in, 3 out]
          }
          frame True {
            n310 = call <vilib>:"Add State to Queue with vData.vi"("queue in"=w909, "state in"="Action: ExecTDMSLogData", "error in"=w907) -> ("error out"=w906:errorcluster)  [unwired: 9 in, 3 out]
          }
        }
      }
      frame "------ Macro ------" {
      }
      frame "Macro: Init" {
        n311 = call-poly <vilib>:"Polymorphic - Add States(s) To Queue.vi"("queue in"=w913, "states in"="Initialize\nIdle", "error in"=w916) -> ("error out"=w914:errorcluster)  [unwired: 10 in, 2 out]
      }
      frame "------ Cmd ------" {
      }
      frame "CMD: OpenTDMSFileRef" {
        # "Just in case. Nominally not required if close logfile was called"
        n312 = Unbundle By Name(w929) -> ("TDMS folder"=w927:path, "tdms fileref"=w931:refnum<k34>)
        n313 = TDMS Close(8:w926, 11:w931) -> (0:w930:errorcluster)  [unwired: 1 out]
        n314 = call <userlib>:"Clear All Errors__ogtk.vi"("Error In"=w930) -> ("Error Out"=w928:errorcluster)  [unwired: 3 in]
        n315 = call "Create TDMS File.vi"("error in (no error)"=w928, "LogFile Folder"=w927) -> ("error out"=w921:errorcluster, "tdms ref"=w924:refnum<k34>, "TDMS File Pathname"=w923:path)  [unwired: 7 in]
        n316 = Bundle By Name(cluster=w929, "TDMS file pathname"=w923, "tdms fileref"=w924) -> (w925:T1)
        n317 = call <vilib>:"Add State to Queue with vData.vi"("queue in"=w919, "state in"="Action: SendStatusMsg >> TDMS File Opened", "error in"=w921) -> ("error out"=w920:errorcluster)  [unwired: 9 in, 3 out]
      }
      frame "CMD: CloseTDMSFileRef" {
        n318 = Unbundle By Name(w937) -> ("TDMSLogging"=w936:bool)
        n319 = case shown="False" w936 {
          tunnel: w940 -> [w946 w955]
          tunnel: [w945 w954] -> w939
          tunnel: w937 -> [w943 w949]
          tunnel: [w942 w949] -> w938
          tunnel: w932 -> [_ w953]
          tunnel: ["Action: SendStatusMsg >> TDMS File Closed" _] -> w935
          frame False {
            n320 = in-place {
              in-place-border: [w948] -> w944
              n321 = in-place-cluster #2(w943) -> ("tdms fileref"=w948)
              n322 = in-place-cluster #2("tdms fileref"=refnum<k0> refnum) -> (w942:cluster{})
            }
            n323 = TDMS Close(8:w946, 11:w944) -> (0:w945:errorcluster)  [unwired: 1 out]
          }
          frame True {
            n324 = call "ReverseStringLines.vi"("Lines in"="CMD: StopTDMSLogging\nCMD: CloseTDMSFileRef" ("states in")) -> ("Reversed Lines out"=w950:string)  [unwired: 4 in]
            n325 = call-poly <vilib>:"Polymorphic - Add States(s) To Queue.vi"("queue in"=w953, "mode (back)"=enum16{"back", "front"}."front", "states in"=w950, "error in"=w955) -> ("error out"=w954:errorcluster)  [unwired: 9 in, 2 out]
          }
        }
        n326 = call <userlib>:"Clear All Errors__ogtk.vi"("Error In"=w939) -> ("Error Out"=w934:errorcluster)  [unwired: 3 in]
        n327 = call <vilib>:"Add State to Queue with vData.vi"("queue in"=w932, "state in"=w935, "error in"=w934) -> ("error out"=w933:errorcluster)  [unwired: 9 in, 3 out]
      }
      frame "CMD: StartTDMSLogging" {
        n328 = Unbundle By Name(w980) -> ("tdms fileref"=w985:refnum<k34>, "Self Reference"=w983:refnum<class "LogEngine.lvclass">, "TDMS file pathname"=w984:path)
        n329 = Unbundle By Name(w980) -> ("SMQ"=w977:refnum<queue>)
        n330 = call "Get Logger State Data.vi"("error in (no error)"=w981, "LogEngine"=w983) -> ("error out"=w959:errorcluster, "Logger State Data"=w982:T7, "LogEngine out"=w961:refnum<class "LogEngine.lvclass">)  [unwired: 7 in]
        n331 = Not A Number/Path/Refnum?(number/path/refnum=w985) -> (NaN/Path/Refnum?=w986:bool)
        n332 = call "Get ObjData.vi"("error in (no error)"=w959, "LogEngine"=w961) -> ("error out"=w958:errorcluster, "Obj Data"=w957:T16, "LogEngine out"=w960:refnum<class "LogEngine.lvclass">)  [unwired: 7 in]
        n333 = Unbundle By Name(w957) -> ("LogHeaderData.SamplingRate"=w956:dbl)
        n334 = case shown="False" w986 {
          tunnel: [w1000 w1008] -> w987
          tunnel: w980 -> [w999 w1008]
          tunnel: w960 -> [w996 _]
          tunnel: w958 -> [w998 w1009]
          tunnel: [w997 w1009] -> w971
          tunnel: w984 -> [w992 _]
          tunnel: w982 -> [w995 w1002]
          tunnel: [TRUE FALSE] -> w979
          tunnel: [w992 path ""] -> w978
          tunnel: ["TDMS Logging Started" "TDMS Logging Stopped"] -> w963
          tunnel: [w990 w1002] -> w962
          tunnel: w956 -> [w988 _]
          frame False {
            w994 = TD_Logger_State--enum."Logging" ("Logger State")
            n335 = Reciprocal(x=w988) -> (1/x=w989:dbl)
            n336 = Bundle By Name(cluster=w995, "TDMS Logging State"=w994, "TDMS File path"=w992) -> (w990:T7)
            n337 = Bundle By Name(cluster=w999, "Sampling dt(s)"=w989, "TDMSLogging"=TRUE ("LocalSMData.Logging"), "Logger State Data.TDMS File path"=w992, "Logger State Data.TDMS Logging State"=w994) -> (w1000:T1)
            n338 = call "Fire LogEngineStateChanged Event_LogEngine.vi"("error in (no error)"=w998, "NEW State Data"=w990, "LogEngine"=w996) -> ("error out"=w997:errorcluster)  [unwired: 7 in, 1 out]
          }
          frame True {
            n339 = call "Dialog Box Timeout v2.vi"("Timeout (s)"=5.0, "Message"="TDMS File Reference is Invalid.\nTDMS File Reference Must Be Opened\nBefore Starting TDMS Logging.") -> ()  [unwired: 9 in, 1 out]
          }
        }
        n340 = Bundle(w979, "Logger State Data"=w962, "TDMS file pathname"=w978) -> (w975:T29)  [unwired: 1 in]
        n341 = call <vilib>:"Add State to Queue with vData.vi"("queue in"=w977, "state in"="Action: UpdateSMData >> TDMSLoggerState", "vData (\"\")"=w975, "error in"=w958) -> ("error out"=w966:errorcluster)  [unwired: 8 in, 3 out]
        n342 = Format Into String(format string="Action: SendStatusMsg >> %s", error in=w966, w963) -> (resulting string=w968:string, error out=w965:errorcluster)  [unwired: 1 in]
        n343 = Bundle("TDMSLoggerState", w975) -> (w973:T30)  [unwired: 1 in]
        n344 = call <vilib>:"Add State to Queue with vData.vi"("queue in"=w967, "state in"=w968, "error in"=w965) -> ("error out"=w969:errorcluster)  [unwired: 9 in, 3 out]
        n345 = property on="localData" class="Clust (strict)"(error in=w969, "Val(Sgnl)"=w973) -> (error out=w970:errorcluster)  [unwired: 1 in, 1 out]
        n346 = Merge Errors(w970, w971) -> (w972:errorcluster)
      }
      frame "CMD: StopTDMSLogging" {
        w1026 = path ""
        w1027 = TD_Logger_State--enum."NotLogging" ("Logger State")
        n347 = Unbundle By Name(w1014) -> ("Self Reference"=w1033:refnum<class "LogEngine.lvclass">)
        n348 = Unbundle By Name(w1014) -> ("SMQ"=w1025:refnum<queue>)
        n349 = call "Get Logger State Data.vi"("error in (no error)"=w1029, "LogEngine"=w1033) -> ("error out"=w1019:errorcluster, "Logger State Data"=w1031:T7, "LogEngine out"=w1032:refnum<class "LogEngine.lvclass">)  [unwired: 7 in]
        n350 = Bundle By Name(cluster=w1031, "TDMS Logging State"=w1027, "TDMS File path"=w1026) -> (w1016:T7)
        n351 = Bundle(FALSE, "Logger State Data"=w1016, path "") -> (w1024:cluster{bool, "Logger State Data":T7, path})  [unwired: 1 in]
        n352 = call <vilib>:"Add State to Queue with vData.vi"("queue in"=w1025, "state in"="Action: UpdateSMData >> TDMSLoggerState", "vData (\"\")"=w1024, "error in"=w1019) -> ("error out"=w1022:errorcluster)  [unwired: 8 in, 3 out]
        n353 = Bundle By Name(cluster=w1014, "TDMSLogging"=FALSE ("LocalSMData.Logging"), "Logger State Data.TDMS File path"=w1026, "Logger State Data.TDMS Logging State"=w1027) -> (w1030:T1)
        n354 = Bundle("TDMSLoggerState", w1024) -> (w1023:T31)  [unwired: 1 in]
        n355 = property on="localData" class="Clust (strict)"(error in=w1022, "Val(Sgnl)"=w1023) -> (error out=w1018:errorcluster)  [unwired: 1 in, 1 out]
        n356 = call "Fire LogEngineStateChanged Event_LogEngine.vi"("error in (no error)"=w1018, "NEW State Data"=w1016, "LogEngine"=w1032) -> ("error out"=w1012:errorcluster)  [unwired: 7 in, 1 out]
        n357 = call <vilib>:"Add State to Queue with vData.vi"("queue in"=w1010, "state in"="Action: SendStatusMsg >> TDMS Logging Stopped", "error in"=w1012) -> ("error out"=w1011:errorcluster)  [unwired: 9 in, 3 out]
      }
      frame "------ Action ------" {
      }
      frame "Action: SendStatusMsg" {
        n358 = Unbundle By Name(w1037) -> ("StatusStr Ref"=w1039:refnum<vi>)
        n359 = call <vilib>:"format status message v2.vi"("status msg"=w1036, "Str Refnum"=w1039) -> ("error out"=w1038:errorcluster)  [unwired: 5 in, 4 out]
        n360 = call <userlib>:"Clear All Errors__ogtk.vi"("Error In"=w1038) -> ()  [unwired: 3 in, 1 out]
      }
      frame "Action: UpdateSMData" {
        n361 = case shown="\"Log&TDMS_Folders\"" w1045 {
          tunnel: w1046 -> [_ w1061 w1071 w1078]
          tunnel: w1042 -> [w1047 w1060 w1070 w1077]
          tunnel: w1044 -> [w1048 w1059 w1069 w1076]
          tunnel: [w1048 w1058 w1068 w1075] -> w1043
          tunnel: [w1047 w1057 w1067 w1073] -> w1041
          frame Default {
          }
          frame "LoggerState" {
            n362 = Bundle(FALSE, "Logger State Data"=T7 {"Logger State"=enum."Unknown", "TDMS Logging State"=enum."Unknown", "LogFile path"=path "", "TDMS File path"=path "", "vData"=variant}, path "") -> (w1054:cluster{bool, "Logger State Data":T7, path})  [unwired: 1 in]
            n363 = Variant To Data(error in=w1060, type=w1054, Variant=w1061) -> (data=w1053:cluster{bool, "Logger State Data":T7, path}, error out=w1057:errorcluster)
            n364 = Unbundle(w1053) -> (w1052:bool, "Logger State Data"=w1051:T7, w1049:path)
            n365 = Bundle By Name(cluster=w1059, "Logging"=w1052, "Logger State Data"=w1051, "LogFile pathname"=w1049) -> (w1058:T1)
          }
          frame "Log&TDMS_Folders" {
            w1063 = path ""
            n366 = Bundle(w1063, w1063) -> (w1062:cluster{path, path})  [unwired: 1 in]
            n367 = Variant To Data(error in=w1070, type=w1062, Variant=w1071) -> (data=w1066:cluster{path, path}, error out=w1067:errorcluster)
            n368 = Unbundle(w1066) -> (w1065:path, w1064:path)
            n369 = Bundle By Name(cluster=w1069, "LogFile folder"=w1065, "TDMS folder"=w1064) -> (w1068:T1)
          }
          frame "SessionSettings" {
            n370 = Variant To Data(error in=w1077, type=T5 {"Job_ID"="", "Operator_ID"="", "Station_ID"="", "Job_Description"=""} ("Session Settings"), Variant=w1078) -> (data=w1074:T5, error out=w1073:errorcluster)
            n371 = Bundle By Name(cluster=w1076, "LogHeaderData.SessionSettings"=w1074) -> (w1075:T1)
          }
        }
      }
      frame "Action: ExecTDMSLogData" {
        # "If TDMSLogging = False,\nThe data Q is flushed.\n\nThis case must be executed\neven if not presently TDMS\nLogging so that Q will not\nexplode in size."
        # "#NOTE: AVC2 app presently has\nonly a single AI task"
        n372 = Unbundle By Name(w1080) -> ("quitting"=w1082:bool, "TDMSLogging"=w1088:bool, "Self Reference"=w1083:refnum<class "LogEngine.lvclass">, "tdms fileref"=w1087:refnum<k34>, "DAQ RawData Q []"=w1086:T2[])
        n373 = Index Array(array=w1086, index=0) -> (element=w1084:T2)
        n374 = Unbundle By Name(w1084) -> ("DAQ RawData Q"=w1081:T3)
        n375 = Unbundle By Name(w1080) -> ("Sampling dt(s)"=w1079:dbl)
        n376 = case shown="False" w1082 {
          tunnel: w1090 -> [w1097 w1098]
          tunnel: [w1096 w1098] -> w1089
          tunnel: w1088 -> [w1095 _]
          tunnel: w1087 -> [w1094 _]
          tunnel: w1081 -> [w1093 _]
          tunnel: w1083 -> [w1092 _]
          tunnel: w1079 -> [w1091 _]
          frame False {
            n377 = call "Write TDMS with Converted RawDataQ ScanData.vi"("dt(s)"=w1091, "Enable TDMS Write"=w1095, "error in (no error)"=w1097, "DAQ RawData Q"=w1093, "tdms ref"=w1094, "LogEngine in"=w1092) -> ("error out"=w1096:errorcluster)  [unwired: 4 in, 1 out]
          }
          frame True {
          }
        }
      }
      frame "Action: FlushRawDataQ" {
        n378 = Unbundle By Name(w1099) -> ("DAQ RawData Q []"=w1100:T2[])
        n379 = for {
          tunnel: w1100 -> [w1105] mode=indexing
          shift-right: [w1106] -> w1102
          shift-left: w1103 -> [w1107]
          n380 = Unbundle(w1105) -> ("DAQ RawData Q"=w1104:T3)  [unwired: 1 out]
          n381 = Flush Queue(queue=w1104, error in (no error)=w1107) -> (error out=w1106:errorcluster)  [unwired: 2 out]
        }
        n382 = call <userlib>:"Clear All Errors__ogtk.vi"("Error In"=w1102) -> ("Error Out"=w1101:errorcluster)  [unwired: 3 in]
      }
      frame "----------- HOLD --------------" {
      }
      frame "HOLD  __CMD: Append TDMS" {
        n383 = disable-structure shown="Enabled" {
          disable-tunnel: [w1123 w1134] -> w1114
          disable-tunnel: w1113 -> [w1121 _]
          disable-tunnel: w1112 -> [w1120 w1135]
          disable-tunnel: [w1116 w1135] -> w1111
          disable-tunnel: w1110 -> [w1115 w1134]
          frame Disabled {
            w1117 = T32 {"Actuator ID"=[], "Cap"=[], "DF"=[], "Parameter"=[], "Parameter label"="", "Notes"=""}  # Post-Sequence Parameters
            n384 = Variant To Data(error in=w1115, type=w1117, Variant=w1121) -> (error out=w1122:errorcluster)  [unwired: 1 out]
            n385 = Unbundle By Name(w1120) -> ("TDMS file pathname"=w1129:path)
            n386 = TDMS Open(8:w1122, 10:T28."open" ("operation (0:open)"), 11:w1129) -> (0:w1124:errorcluster, 3:w1127:refnum<k34>)  [unwired: 4 in]
            n387 = TDMS Set Properties(5:variant[] [] ("property values"), 7:string[] [] ("property names"), 8:w1124, 10:"Post Sequence Parameters" ("group name"), 11:w1127) -> (0:w1125:errorcluster, 3:w1126:refnum<k34>)  [unwired: 1 in, 2 out]
            n388 = disable-structure shown="Disabled" {
              disable-tunnel: w1120 -> [w1132 w1133]
              disable-tunnel: [w1131 w1133] -> w1116
              frame Disabled {
                n389 = Bundle By Name(cluster=w1132) -> (w1131:T1)  [unwired: 1 in]
              }
              frame Enabled {
              }
            }
            n390 = TDMS Close(8:w1125, 11:w1126) -> (0:w1123:errorcluster)  [unwired: 1 out]
          }
          frame Enabled {
          }
        }
      }
    }
  }
  n391 = Merge Errors(w11, w10, w4) -> (w3:errorcluster)
  n392 = flat-sequence {
    tunnel: w3 -> [w1141]
    tunnel: [w1136] -> w2
    tunnel: w1 -> [w1150]
    frame #0 {
      n393 = Unbundle By Name(w1150) -> ("Core.process sync notifier"=w1148:refnum<notifier>, "SMQ"=w1146:refnum<queue>, "TDMS SMQ"=w1144:refnum<queue>)
      n394 = call <userlib>:"Clear All Errors__ogtk.vi"("Error In"=w1141) -> ("Error Out"=w1138:errorcluster)  [unwired: 3 in]
      n395 = Release Queue(queue=w1144, force destroy? (F)=TRUE, error in (no error)=w1138) -> (error out=w1143:errorcluster)  [unwired: 2 out]
      n396 = call <userlib>:"Clear All Errors__ogtk.vi"("Error In"=w1143) -> ("Error Out"=w1139:errorcluster)  [unwired: 3 in]
      n397 = Release Queue(queue=w1146, force destroy? (F)=TRUE, error in (no error)=w1139) -> (error out=w1142:errorcluster)  [unwired: 2 out]
      n398 = call <userlib>:"Clear All Errors__ogtk.vi"("Error In"=w1142) -> ("Error Out"=w1140:errorcluster)  [unwired: 3 in]
      n399 = Send Notification(notification=TRUE, notifier=w1148, error in (no error)=w1140) -> (error out=w1137:errorcluster)  [unwired: 1 out]
      n400 = call <userlib>:"Clear All Errors__ogtk.vi"("Error In"=w1137) -> ("Error Out"=w1136:errorcluster)  [unwired: 3 in]
    }
  }
  "error out" <- w2
